vi "ref_Wrist_imp_PYBR_CH_v9.vi"() -> ()   [LabVIEW 2017]
uses:
  <vilib>/rvi/FXPMathLib/FxpSinAndCos/subVIs/nifxpmath_SinAndCos_SimConfig.ctl
  <vilib>/rvi/Emulation/niFpgaGetClockAttributes.vi
  <vilib>/rvi/Emulation/niFpgaSctlEmulationGetInTimedLoop.vi
  <vilib>/rvi/Emulation/niFpgaEmulationReportErrorSimple.vi
  <vilib>/rvi/eio/common/nirviEmuTemplateMethod_errors.vi
  <vilib>/rvi/Emulation/niFpgaProcessEmulError.vi
  <vilib>/rvi/Emulation/niFpgaCriticalErrorInLSC.vi
  <vilib>/rvi/interface/RandomDataEmulation/nirviRandomDataMultiElementFPGAFIFO.vi
  <instcachedir>/0/nirviRandomDataMultiElementFPGAFIFO_6740B454F3C245F78F76ED91F73FD8DB.lvgen/nirviRandomDataMultiElementFPGAFIFO_6740B454F3C245F78F76ED91F73FD8DB_003.vi
  <vilib>/rvi/interface/RandomDataEmulation/niFpgaRandomDataHandleErrors.vi
  <vilib>/rvi/FXPMathLib/FxpSinAndCos/simVIs/DllFxpSinAndCosTemp_sub.vi
  <vilib>/eio/EIONode/EIONode.xnode
  <vilib>/rvi/FXPMathLib/FxpMul/XNode/nifxpmath_Multiplier.xnode
  <vilib>/rvi/FXPMathLib/FxpSub/XNode/nifxpmath_Sub.xnode
  <vilib>/rvi/FXPMathLib/FxpAdd/XNode/nifxpmath_Add.xnode
  <vilib>/rvi/DataTransferAndStorage/Container/XNode/niFpgaContainer.xnode
  <vilib>/rvi/interface/RandomDataEmulation/nirviRandomDataFpgaMultiElementTemplate.vi
  <vilib>/rvi/FXPMathLib/FxpSinAndCos/XNode/nifxpmath_SinAndCos.xnode
  <vilib>/rvi/Analysis/measure/butterworth/XNode/niFpgaButterworthFilter.xnode
  <vilib>/rvi/FXPMathLib/sim/FxpSim.dll
panel:
  in  "Start_two":bool=TRUE
  in  "FIFO":i16(ring) items=["Inverse", "Forward", "Elbow"]
  out "Db_e":fxp<+/-,26,11>
  in  "time stop b":fxp<+,64,32>=5.0 format="%#_42g"
  out "Forward/Backward (b)":bool
  in  "CASE (b)":i16(ring) caption="Numeric" items=["Backward", "Forward", "Original"]
  in  "Sin/Step (b)":i16(ring) items=["Step", "Sin"]
  in  "ATOM b\nVelocity method":i16(ring) items=["M_average", "T_method"]
  in  "Encoder b\nVelocity method":i16(ring) items=["M_average", "T_method"]
  in  "phase(rad/pi)_b":fxp<+/-,16,3>
  in  "ATOM (P/Y)\nVelocity Method":i16(ring) items=["M_Average", "T_method"]
  in  "Encoder (P/Y)\nVelocity Method":i16(ring) items=["M_average", "T_method"]
  out "Encoder Position_b":i32
  out "rad(NrTheta)_b":fxp<+/-,33,18> format="%.21g"
  out "Db(mm)":fxp<+/-,22,7>
  in  "Encoder Reset_b":bool
  out "vd_b_F":fxp<+/-,20,5>
  out "vq_b_F":fxp<+/-,20,5> format="%.57g"
  out "Fb_PID":fxp<+/-,21,11>
  in  "fb_tolerance":fxp<+,32,9>=1.0
  out "fb_tilde":fxp<+/-,21,11>
  in  "Kpb":fxp<+,11,7>=0.375
  in  "Kib":fxp<+,27,10>
  in  "Kdb":fxp<+,26,2>
  out "fbt_i":fxp<+/-,32,9>
  out "dFb_PID":fxp<+/-,25,15>
  in  "scaled coe_dFb_PID":i32[](array[numeric])=[1067016412, 3362706]
  out "Db_dd":fxp<+/-,25,15>
  in  "scaled coe_Db_dd":i32[](array[numeric])=[1067016412, 3362706]
  out "xb_dd":fxp<+/-,25,15>
  in  "scaled coe_xb_dd":i32[](array[numeric])=[1067016412, 3362706]
  in  "kb":fxp<+,15,8>
  out "xb(mm)":fxp<+/-,22,7>
  out "fb":fxp<+/-,20,10>
  in  "Atom Reset_b":bool
  out "Atom_Position_b":i32
  out "Sin wave time (s) b":fxp<+,64,32>
  out "Db_d(mm/s)":fxp<+/-,32,12>
  out "Omega_b(rad/s)":fxp<+/-,32,18>
  in  "xb_d_M_avg_Tc (uSec)":u32 caption="M_avg_Tc (uSec)"
  out "xb_d(M_avg method)":fxp<+/-,25,10>
  out "vb_b":fxp<+/-,20,5> format="%.21g"
  out "va_b":fxp<+/-,20,5> format="%.21g"
  in  "Stop Motor_b":bool
  out "Dabr_sin/cos":fxp<+/-,22,8>
  in  "Sin_offset_b":fxp<+/-,16,5>
  in  "Sin_mag_b":fxp<+/-,17,6>
  out "Dabr_d":fxp<+/-,33,10>
  out "Dabr_dd":fxp<+/-,34,12>
  in  "Sin_freq_b (Hz)":fxp<+,16,3>
  out "fbr":fxp<+/-,20,10>
  in  "Kvb":fxp<+,15,8>
  in  "Bvb":fxp<+,15,8>
  in  "Dbr":fxp<+/-,22,8>
  out "Step/Sin Db":bool
  out "fbt_d":fxp<+/-,25,15>
  out "Dab_ed":fxp<+/-,33,10>
  out "Dab_edd":fxp<+/-,34,12>
  out "xb_d(mm/s)":fxp<+/-,25,10>
  in  "Db_d_M_avg_Tc (uSec)":u32 caption="M_avg_Tc (uSec)"
  out "Omega_b(M_avg)":fxp<+/-,32,18>
  out "Db_d(M_avg method)":fxp<+/-,32,12>
  in  "fb_lmpact":fxp<+,16,11>
  in  "Step / Sin (py)":i16(ring) items=["Step", "Sin"]
  in  "CASE (py)":i16(ring) caption="Numeric" items=["Backward", "Forward", "Original"]
  out "Dyr_sin/cos":fxp<+/-,24,10>
  in  "Sin_offset_y1":fxp<+/-,16,5>
  in  "Sin_mag_y1":fxp<+/-,17,6>
  out "Dyr_d":fxp<+/-,35,12>
  out "Dyr_dd":fxp<+/-,36,14>
  in  "Sin_freq(Hz)_y1":fxp<+,16,3>
  in  "phase(rad/pi)_y1":fxp<+/-,16,3>
  in  "Sin_offset_y2":fxp<+/-,16,5>
  in  "Sin_mag_y2":fxp<+/-,17,6>
  in  "Sin_freq(Hz)_y2":fxp<+,16,3>
  in  "phase(rad/pi)_y2":fxp<+/-,16,3>
  in  "Sin_offset_y3":fxp<+/-,16,5>
  in  "Sin_mag_y3":fxp<+/-,17,6>
  in  "Sin_freq(Hz)_y3":fxp<+,16,3>
  in  "phase(rad/pi)_y3":fxp<+/-,16,3>
  out "Dy_ed":fxp<+/-,33,10>
  out "Dy_edd":fxp<+/-,34,12>
  out "fyt_d":fxp<+/-,25,15>
  in  "ky":fxp<+,15,8>
  out "Dy_d(mm/s)":fxp<+/-,32,12>
  out "Omega_y(rad/s)":fxp<+/-,32,18>
  out "xy_d(mm/s)":fxp<+/-,25,10>
  out "xy_d(M_avg)":fxp<+/-,25,10>
  out "Omega_y(M_avg)":fxp<+/-,32,18>
  out "Dy_d(M_avg)":fxp<+/-,32,12>
  out "Encoder Position_y":i32
  out "rad(NrTheta)_y":fxp<+/-,33,18> format="%.21g"
  out "Dy(mm)":fxp<+/-,22,7>
  out "vd_y_F":fxp<+/-,20,5>
  out "vq_y_F":fxp<+/-,20,5> format="%.57g"
  out "Fy_PID":fxp<+/-,21,11>
  in  "fy_tolerance":fxp<+,32,9>=1.0
  out "fy_tilde":fxp<+/-,21,11>
  in  "Kpy":fxp<+,11,7>=0.375
  in  "Kiy":fxp<+,27,10>
  in  "Kdy":fxp<+,26,2>
  out "fyt_i":fxp<+/-,32,9>
  out "dFy_PID":fxp<+/-,25,15>
  out "Dy_dd":fxp<+/-,25,15>
  out "xy_dd":fxp<+/-,25,15>
  out "xy(mm)":fxp<+/-,22,7>
  out "fy":fxp<+/-,20,10>
  out "Atom_Position_y":i32
  out "vb_y":fxp<+/-,20,5> format="%.21g"
  out "va_y":fxp<+/-,20,5> format="%.21g"
  out "fyr":fxp<+/-,20,10>
  in  "Kvy":fxp<+,15,8>
  in  "Bvy":fxp<+,10,3>
  out "Dy_e":fxp<+/-,26,11>
  in  "Dyr":fxp<+/-,22,8>
  out "Forward/Backward (py)":bool
  in  "time stop py":fxp<+,64,32>=5.0 format="%#_42g"
  in  "Sin_offset_p3":fxp<+/-,16,5>
  in  "Sin_mag_p3":fxp<+/-,17,6>
  in  "Sin_freq(Hz)_p3":fxp<+,16,3>
  in  "phase(rad/pi)_p3":fxp<+/-,16,3>
  in  "Sin_offset_p2":fxp<+/-,16,5>
  in  "Sin_mag_p2":fxp<+/-,17,6>
  in  "Sin_freq(Hz)_p2":fxp<+,16,3>
  in  "phase(rad/pi)_p2":fxp<+/-,16,3>
  in  "phase(rad/pi)_p1":fxp<+/-,16,3>
  in  "fpy_Impact":fxp<+,16,11>
  in  "Dpy_d_M_avg_Tc (uSec)":u32 caption="M_avg_Tc (uSec)"
  out "Omega_p(rad/s)":fxp<+/-,32,18>
  out "Omega_p(M_avg)":fxp<+/-,32,18>
  out "xp_dd":fxp<+/-,25,15>
  in  "scaled coe_xpy_dd":i32[](array[numeric])=[1067016412, 3362706]
  out "Dp_dd":fxp<+/-,25,15>
  in  "scaled coe_Dpy_dd":i32[](array[numeric])=[1067016412, 3362706]
  out "Dp_edd":fxp<+/-,34,12>
  out "Dp_ed":fxp<+/-,33,10>
  out "fpr":fxp<+/-,20,10>
  in  "Kvp":fxp<+,15,8>
  in  "Bvp":fxp<+,10,3>
  out "Dp_e":fxp<+/-,26,11>
  in  "Dpr":fxp<+/-,22,8>
  out "Step/Sin Dpy":bool
  out "Dpr_sin/cos":fxp<+/-,24,10>
  in  "Sin_offset_p1":fxp<+/-,16,5>
  in  "Sin_mag_p1":fxp<+/-,17,6>
  out "Dpr_d":fxp<+/-,35,12>
  out "Dpr_dd":fxp<+/-,36,14> format="%.26g"
  in  "Sin_freq(Hz)_p1":fxp<+,16,3>
  out "Dp_d(M_avg)":fxp<+/-,32,12>
  out "xp_d(M_avg)":fxp<+/-,25,10>
  in  "xpy_d_M_avg_Tc (uSec)":u32 caption="M_avg_Tc (uSec)"
  out "fpt_d":fxp<+/-,25,15>
  out "Dp_d(mm/s)":fxp<+/-,32,12>
  out "Atom_Position_p":i32
  out "xp_d(mm/s)":fxp<+/-,25,10>
  in  "dFb_PID_add":bool
  in  "scaled coe_dFpy_PID":i32[](array[numeric])=[1067016412, 3362706]
  out "dFp_PID":fxp<+/-,25,15>
  out "Sin wave time (s)":fxp<+,64,32>
  in  "Atom Reset":bool
  out "xp(mm)":fxp<+/-,22,7>
  in  "Coe Ini":bool
  in  "Encoder Reset":bool
  in  "Stop Motor":bool
  in  "Kip":fxp<+,27,10>
  in  "Kdp":fxp<+,26,2>
  out "fpt_i":fxp<+/-,32,9>
  in  "Kpp":fxp<+,11,7>=0.375
  in  "kp":fxp<+,15,8>
  out "fp":fxp<+/-,20,10>
  out "fp_tilde":fxp<+/-,21,11>
  out "Fp_PID":fxp<+/-,21,11>
  in  "fp_tolerance":fxp<+,32,9>=1.0
  out "Encoder Position_p":i32
  out "rad(NrTheta)_p":fxp<+/-,33,18> format="%.21g"
  out "Dp(mm)":fxp<+/-,22,7>
  out "vq_p_F":fxp<+/-,20,5> format="%.57g"
  out "vd_p_F":fxp<+/-,20,5>
  out "va_p":fxp<+/-,20,5> format="%.21g"
  out "vb_p":fxp<+/-,20,5> format="%.21g"
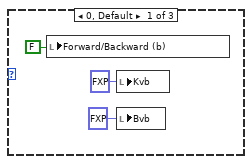
[diagram p4: hidden frame]
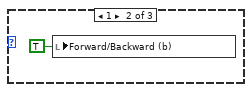
[diagram p5: hidden frame]
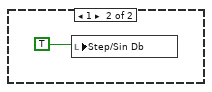
[diagram p6: hidden frame]
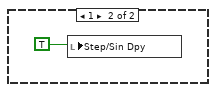
[diagram p7: hidden frame]
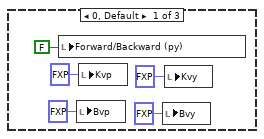
[diagram p8: hidden frame]
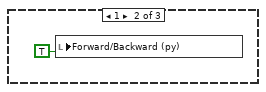
[diagram p9: hidden frame]
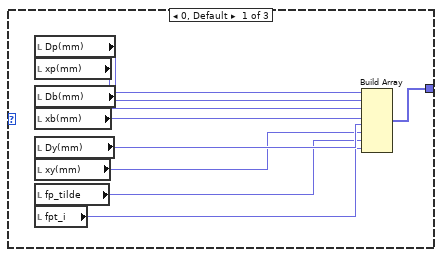
[diagram p20: hidden frame]
diagram:
  w2 = FALSE ("Encoder Reset_b")
  w11 = 25  # M_avg_n
  w7 = 25  # M_avg_n
  w21 = 25  # M_avg_n
  w17 = 25  # M_avg_n
  w1 = FALSE ("Atom Reset_b")
  w5 = TRUE ("Stop Motor_b")
  w26 = 25  # M_avg_n
  w30 = 25  # M_avg_n
  n1 = for {
    N: w11 -> [_]
    tunnel: [w34] -> w13 mode=indexing
    tunnel: [w32] -> w12 mode=indexing
    tunnel: ["Db_d_M_avg_Tc (uSec)"] -> w10
    n2 = local read "Encoder Position_b"() -> (w32:i32)
    n3 = call "Wait11"("Count(uSec)"="Db_d_M_avg_Tc (uSec)") -> ("Tick Count(uSec)"=w34:u32)
  }
  n4 = for {
    N: w7 -> [_]
    tunnel: [w37] -> w6 mode=indexing
    tunnel: ["xb_d_M_avg_Tc (uSec)"] -> w8
    tunnel: [w35] -> w9 mode=indexing
    n5 = local read "Atom_Position_b"() -> (w35:i32)
    n6 = call "Wait9"("Count(uSec)"="xb_d_M_avg_Tc (uSec)") -> ("Tick Count(uSec)"=w37:u32)
  }
  n7 = while "Db_d(M_avg method)" {
    shift-right: [w48] -> _
    shift-left: w13 -> [w51]
    tunnel: w11 -> [w49]
    shift-right: [w46] -> _
    shift-left: w12 -> [w44]
    shift-right: [w39] -> _
    shift-left: _ -> [w42]
    tunnel: w10 -> [w41]
    stop <- FALSE stop-if-true
    n8 = Index Array(array=w51, index=0) -> (element=w47:u32)
    n9 = Multiply(x=w49, y=w41) -> (x*y=w54:u32)
    n10 = Index Array(array=w44, index=0) -> (element=w43:i32)
    n11 = Add(x=w54, y=w47) -> (x+y=w53:u32)
    n12 = call "Tick Count20"() -> ("Tick Count(uSec)"=w50:u32)
    n13 = Greater Or Equal?(x=w50, y=w53) -> (x >= y?=w52:bool)
    n14 = case shown="True" w52 {
      tunnel: w51 -> [w59 w81]
      tunnel: w50 -> [_ w75]
      tunnel: w49 -> [_ w64]
      tunnel: [w59 w77] -> w48
      tunnel: w47 -> [_ w76]
      tunnel: w44 -> [w58 w65]
      tunnel: [w58 w63] -> w46
      tunnel: [w57 w62] -> w39
      tunnel: w43 -> [_ w60]
      tunnel: w42 -> [w57 _]
      frame False {
      }
      frame True {
        n15 = local read "Encoder Position_b"() -> (w69:i32)
        n16 = Subtract(x=w75, y=w76) -> (x-y=w74:u32)
        n17 = To Fixed-Point(number=w74) -> (fixed-point=w61:fxp<+,32,32>)  [unwired: 1 in]
        n18 = Insert Into Array(array=w81, index=w64, new element=w75) -> (w80:u32[])
        n19 = Insert Into Array(array=w65, index=w64, new element=w69) -> (w66:i32[])
        n20 = Subtract(x=w69, y=w60) -> (x-y=w70:i32)
        n21 = Multiply(x=w70, y=2500) -> (x*y=w72:i32)
        n22 = Delete From Array(array=w80, length=1, index=0) -> (array with subset deleted=w77:u32[])  [unwired: 1 out]
        n23 = Delete From Array(array=w66, length=1, index=0) -> (array with subset deleted=w63:i32[])  [unwired: 1 out]
        n24 = To Fixed-Point(number=w72) -> (fixed-point=w73:fxp<+/-,32,32>)  [unwired: 1 in]
        n25 = Divide(x=w73, y=w61) -> (x/y=w62:fxp<+/-,32,12>)
      }
    }
    "Db_d(M_avg method)" <- w39
    n26 = Multiply(x=w39, y=fxp<+/-,32,12> 3.1415929794311523 ("x")) -> (x*y=→"Omega_b(M_avg)":fxp<+/-,32,18>)
  }
  n27 = while "M_avg method" {
    shift-right: [w89] -> _
    shift-left: w6 -> [w92]
    shift-right: [w83] -> _
    shift-left: w9 -> [w86]
    tunnel: w7 -> [w90]
    shift-right: [w85] -> _
    shift-left: _ -> [w84]
    tunnel: w8 -> [w82]
    stop <- FALSE stop-if-true
    n28 = Index Array(array=w92, index=0) -> (element=w88:u32)
    n29 = Multiply(x=w90, y=w82) -> (x*y=w95:u32)
    n30 = Index Array(array=w86, index=0) -> (element=w87:i32)
    n31 = Add(x=w95, y=w88) -> (x+y=w94:u32)
    n32 = call "Tick Count18"() -> ("Tick Count(uSec)"=w91:u32)
    n33 = Greater Or Equal?(x=w91, y=w94) -> (x >= y?=w93:bool)
    n34 = case shown="True" w93 {
      tunnel: w92 -> [w101 w123]
      tunnel: w91 -> [_ w117]
      tunnel: w90 -> [_ w103]
      tunnel: [w101 w119] -> w89
      tunnel: w88 -> [_ w118]
      tunnel: w86 -> [w100 w114]
      tunnel: w87 -> [_ w110]
      tunnel: [w99 w105] -> w85
      tunnel: w84 -> [w99 _]
      tunnel: [w100 w104] -> w83
      frame False {
      }
      frame True {
        n35 = local read "Atom_Position_b"() -> (w111:i32)
        n36 = Subtract(x=w117, y=w118) -> (x-y=w116:u32)
        n37 = To Fixed-Point(number=w116) -> (fixed-point=w102:fxp<+,32,32>)  [unwired: 1 in]
        n38 = Insert Into Array(array=w123, index=w103, new element=w117) -> (w122:u32[])
        n39 = Insert Into Array(array=w114, index=w103, new element=w111) -> (w115:i32[])
        n40 = Subtract(x=w111, y=w110) -> (x-y=w109:i32)
        n41 = Multiply(x=w109, y=-1000) -> (x*y=w107:i32)
        n42 = Delete From Array(array=w122, length=1, index=0) -> (array with subset deleted=w119:u32[])  [unwired: 1 out]
        n43 = Delete From Array(array=w115, length=1, index=0) -> (array with subset deleted=w104:i32[])  [unwired: 1 out]
        n44 = To Fixed-Point(number=w107) -> (fixed-point=w106:fxp<+/-,32,32>)  [unwired: 1 in]
        n45 = Divide(x=w106, y=w102) -> (x/y=w105:fxp<+/-,25,10>)
      }
    }
    "xb_d(M_avg method)" <- w85
  }
  n46 = while "Encoder_b" {
    shift-right: [w125] -> _
    shift-left: _ -> [w137]
    shift-right: [w124] -> _
    shift-left: _ -> [w136]
    shift-right: [w129] -> _
    shift-left: _ -> [w135]
    stop <- FALSE stop-if-true
    n47 = xnode "FPGA I/O Node"() -> ("Mod4/DI3"=w127:bool, "Mod4/DI4"=w126:bool)  [unwired: 2 in, 2 out]
    n48 = call "encoder_sub.vi"("A_pre"=w137, "B_pre"=w136, "Encoder Position_pre"=w135, "A input"=w127, "Encoder Position Reset"="Encoder Reset_b", "B input"=w126) -> ("A"=w125:bool, "B"=w124:bool, "Encoder Position (Counts)"=w129:i32)  [unwired: 19 in]
    "Encoder Position_b" <- w129
    n49 = To Fixed-Point(number=w129) -> (fixed-point=w132:fxp<+/-,18,18>)  [unwired: 1 in]
    n50 = xnode ("High Throughput Multiply")("x"=w132, "y"=fxp<+/-,15,-7> 0.0012500286102294922) -> ("x*y"=→"Db(mm)":fxp<+/-,22,7>)
    n51 = xnode ("High Throughput Multiply")("x"=w132, "y"=fxp<+,24,0> 0.125) -> ("x*y"=→"rad(NrTheta)_b":fxp<+/-,33,18>)
  }
  n52 = while "Atom_b" {
    shift-right: [w152] -> _
    shift-left: _ -> [w150]
    shift-right: [w151] -> _
    shift-left: _ -> [w149]
    shift-right: [w140] -> _
    shift-left: _ -> [w146]
    stop <- FALSE stop-if-true
    n53 = xnode "FPGA I/O Node"() -> ("Mod4/DI0"=w148:bool, "Mod4/DI1"=w147:bool)  [unwired: 2 in, 2 out]
    n54 = call "encoder_sub.vi"("A_pre"=w150, "B_pre"=w149, "Encoder Position_pre"=w146, "A input"=w148, "Encoder Position Reset"="Atom Reset_b", "B input"=w147) -> ("A"=w152:bool, "B"=w151:bool, "Encoder Position (Counts)"=w140:i32)  [unwired: 19 in]
    "Atom_Position_b" <- w140
    n55 = To Fixed-Point(number=w140) -> (fixed-point=w144:fxp<+/-,18,18>)  [unwired: 1 in]
    n56 = xnode ("High Throughput Multiply")("x"=w144, "y"=fxp<+/-,20,-5> -0.0009999871253967285) -> ("x*y"=w142:fxp<+/-,22,7>)
    "xb(mm)" <- w142
    n57 = Multiply(x=w142, y="kb") -> (x*y=→"fb":fxp<+/-,20,10>)
  }
  n58 = for {
    N: w21 -> [_]
    tunnel: [w156] -> w23 mode=indexing
    tunnel: [w155] -> w22 mode=indexing
    tunnel: [w154] -> w20
    n59 = local read "Dpy_d_M_avg_Tc (uSec)"() -> (w154:u32)
    n60 = local read "Encoder Position_y"() -> (w155:i32)
    n61 = call "Wait7"("Count(uSec)"=w154) -> ("Tick Count(uSec)"=w156:u32)
  }
  n62 = for {
    N: w17 -> [_]
    tunnel: [w159] -> w16 mode=indexing
    tunnel: [w157] -> w18
    tunnel: [w158] -> w19 mode=indexing
    n63 = local read "xpy_d_M_avg_Tc (uSec)"() -> (w157:u32)
    n64 = local read "Atom_Position_y"() -> (w158:i32)
    n65 = call "Wait6"("Count(uSec)"=w157) -> ("Tick Count(uSec)"=w159:u32)
  }
  n66 = for {
    N: w26 -> [_]
    tunnel: [w162] -> w24 mode=indexing
    tunnel: [w160] -> w25 mode=indexing
    tunnel: ["Dpy_d_M_avg_Tc (uSec)"] -> w27
    n67 = local read "Encoder Position_p"() -> (w160:i32)
    n68 = call "Wait4"("Count(uSec)"="Dpy_d_M_avg_Tc (uSec)") -> ("Tick Count(uSec)"=w162:u32)
  }
  n69 = for {
    N: w30 -> [_]
    tunnel: [w165] -> w31 mode=indexing
    tunnel: ["xpy_d_M_avg_Tc (uSec)"] -> w29
    tunnel: [w163] -> w28 mode=indexing
    n70 = local read "Atom_Position_p"() -> (w163:i32)
    n71 = call "Wait3"("Count(uSec)"="xpy_d_M_avg_Tc (uSec)") -> ("Tick Count(uSec)"=w165:u32)
  }
  n72 = while "PID force controller_imp_p" {
    stop <- FALSE stop-if-true
    n73 = flat-sequence {
      tunnel: [w169] -> w166
      tunnel: [w184] -> w167
      tunnel: w166 -> [w183]
      tunnel: w167 -> [w201]
      frame #0 {
        # "SEA imp position controller_p"
        n74 = local read "Step/Sin Dpy"() -> (w182:bool)
        n75 = local read "Dpr_sin/cos"() -> (w181:fxp<+/-,24,10>)
        n76 = local read "Dp(mm)"() -> (w174:fxp<+/-,22,7>)
        n77 = local read "xp(mm)"() -> (w173:fxp<+/-,22,7>)
        n78 = local read "Dp_ed"() -> (w176:fxp<+/-,33,10>)
        n79 = Select(t=w181, s=w182, f="Dpr") -> (s? t:f=w179:fxp<+/-,24,10>)
        n80 = Subtract(x=w174, y=w173) -> (x-y=w175:fxp<+/-,22,7>)
        n81 = Subtract(x=w179, y=w175) -> (x-y=w170:fxp<+/-,25,10>)
        "Dp_e" <- w170
        n82 = Multiply(x=w170, y="Kvp") -> (x*y=w172:fxp<+/-,40,18>)
        n83 = Multiply(x=w176, y="Bvp") -> (x*y=w171:fxp<+/-,43,13>)
        n84 = Add(x=w172, y=w171) -> (x+y=w169:fxp<+/-,20,10>)
        "fpr" <- w169
      }
      frame #1 {
        # "PID force controller_imp_p"
        n85 = local read "fp"() -> (w195:fxp<+/-,20,10>)
        n86 = local read "fpt_d"() -> (w186:fxp<+/-,25,15>)
        n87 = xnode "High Throughput Subtract"("x"=w183, "y"=w195) -> ("x-y"=w197:fxp<+/-,21,11>)
        "fp_tilde" <- w197
        n88 = local read "fpt_i"() -> (w193:fxp<+/-,32,9>)
        n89 = Absolute Value(x=w197) -> (abs(x)=w199:fxp<+,21,11>)
        n90 = xnode ("High Throughput Multiply")("x"="Kpp", "y"=w197) -> ("x*y"=w196:fxp<+/-,33,17>)
        n91 = xnode ("High Throughput Multiply")("x"="Kdp", "y"=w186) -> ("x*y"=w190:fxp<+/-,31,21>)
        n92 = xnode ("High Throughput Add")("x"=w196, "y"=w190) -> ("x+y"=w194:fxp<+/-,21,11>)
        n93 = xnode ("High Throughput Multiply")("x"="Kip", "y"=w193) -> ("x*y"=w192:fxp<+/-,31,14>)
        n94 = Greater?(x=w199, y="fp_tolerance") -> (0:w198:bool)
        n95 = xnode ("High Throughput Add")("x"=w194, "y"=w192) -> ("x+y"=w191:fxp<+/-,21,11>)
        n96 = Select(t=w191, s=w198, f=fxp<+/-,21,11> 0.0) -> (s? t:f=w184:fxp<+/-,21,11>)
        "Fp_PID" <- w184
      }
      frame #2 {
        w204 = fxp<+,3,2> 0.5  # belt_coe
        # "Quadrature drive_p"
        n97 = local read "Omega_p(rad/s)"() -> (w206:fxp<+/-,32,18>)
        n98 = local read "dFp_PID"() -> (w210:fxp<+/-,25,15>)
        n99 = Select(t=fxp<+/-,25,15> 0.0 ("f"), s="dFb_PID_add", f=w210) -> (s? t:f=w207:fxp<+/-,25,15>)
        n100 = Multiply(x=w204, y=w201) -> (x*y=w205:fxp<+/-,24,13>)
        n101 = call "Oriental_step_motor_PKP214D06A.vi"("F_Threshold"=fxp<+,12,12> 10.0, "dFmr"=w207, "omega"=w206, "Fmr"=w205) -> ("vq_F"=→"vq_p_F":fxp<+/-,20,5>, "vd_F"=→"vd_p_F":fxp<+/-,20,5>)  [unwired: 6 in]
      }
    }
  }
  n102 = while "PID force controller_imp_y" {
    stop <- FALSE stop-if-true
    n103 = flat-sequence {
      tunnel: [w215] -> w213
      tunnel: w213 -> [w230]
      tunnel: [w229] -> w212
      tunnel: w212 -> [w247]
      frame #0 {
        # "SEA imp position controller_y"
        n104 = local read "Step/Sin Dpy"() -> (w216:bool)
        n105 = local read "Dyr_sin/cos"() -> (w217:fxp<+/-,24,10>)
        n106 = local read "Dy(mm)"() -> (w224:fxp<+/-,22,7>)
        n107 = local read "xy(mm)"() -> (w225:fxp<+/-,22,7>)
        n108 = local read "Dp_ed"() -> (w222:fxp<+/-,33,10>)
        n109 = Select(t=w217, s=w216, f="Dyr") -> (s? t:f=w219:fxp<+/-,24,10>)
        n110 = Subtract(x=w224, y=w225) -> (x-y=w223:fxp<+/-,22,7>)
        n111 = Subtract(x=w219, y=w223) -> (x-y=w228:fxp<+/-,25,10>)
        "Dy_e" <- w228
        n112 = Multiply(x=w228, y="Kvy") -> (x*y=w226:fxp<+/-,40,18>)
        n113 = Multiply(x=w222, y="Bvy") -> (x*y=w227:fxp<+/-,43,13>)
        n114 = Add(x=w226, y=w227) -> (x+y=w215:fxp<+/-,20,10>)
        "fyr" <- w215
      }
      frame #1 {
        # "PID force controller_imp_y"
        n115 = local read "fy"() -> (w241:fxp<+/-,20,10>)
        n116 = local read "fyt_d"() -> (w232:fxp<+/-,25,15>)
        n117 = xnode "High Throughput Subtract"("x"=w230, "y"=w241) -> ("x-y"=w243:fxp<+/-,21,11>)
        "fy_tilde" <- w243
        n118 = local read "fyt_i"() -> (w239:fxp<+/-,32,9>)
        n119 = Absolute Value(x=w243) -> (abs(x)=w245:fxp<+,21,11>)
        n120 = xnode ("High Throughput Multiply")("x"="Kpy", "y"=w243) -> ("x*y"=w242:fxp<+/-,33,17>)
        n121 = xnode ("High Throughput Multiply")("x"="Kdy", "y"=w232) -> ("x*y"=w236:fxp<+/-,31,21>)
        n122 = xnode ("High Throughput Add")("x"=w242, "y"=w236) -> ("x+y"=w240:fxp<+/-,21,11>)
        n123 = xnode ("High Throughput Multiply")("x"="Kiy", "y"=w239) -> ("x*y"=w238:fxp<+/-,31,14>)
        n124 = Greater?(x=w245, y="fy_tolerance") -> (0:w244:bool)
        n125 = xnode ("High Throughput Add")("x"=w240, "y"=w238) -> ("x+y"=w237:fxp<+/-,21,11>)
        n126 = Select(t=w237, s=w244, f=fxp<+/-,21,11> 0.0) -> (s? t:f=w229:fxp<+/-,21,11>)
        "Fy_PID" <- w229
      }
      frame #2 {
        w250 = fxp<+,3,2> 0.5  # belt_coe
        # "Quadrature drive_y"
        n127 = local read "dFb_PID_add"() -> (w257:bool)
        n128 = local read "Omega_y(rad/s)"() -> (w255:fxp<+/-,32,18>)
        n129 = local read "dFy_PID"() -> (w251:fxp<+/-,25,15>)
        n130 = Select(t=fxp<+/-,25,15> 0.0 ("f"), s=w257, f=w251) -> (s? t:f=w254:fxp<+/-,25,15>)
        n131 = Multiply(x=w250, y=w247) -> (x*y=w256:fxp<+/-,24,13>)
        n132 = call "Oriental_step_motor_PKP214D06A.vi"("F_Threshold"=fxp<+,12,12> 10.0, "dFmr"=w254, "omega"=w255, "Fmr"=w256) -> ("vq_F"=→"vq_y_F":fxp<+/-,20,5>, "vd_F"=→"vd_y_F":fxp<+/-,20,5>)  [unwired: 6 in]
      }
    }
  }
  n133 = while "PID force controller_imp_b" {
    stop <- FALSE stop-if-true
    n134 = flat-sequence {
      tunnel: [w261] -> w258
      tunnel: [w276] -> w259
      tunnel: w258 -> [w275]
      tunnel: w259 -> [w293]
      frame #0 {
        # "SEA imp position controller_b"
        n135 = local read "Step/Sin Db"() -> (w273:bool)
        n136 = local read "Dabr_sin/cos"() -> (w272:fxp<+/-,22,8>)
        n137 = local read "Db(mm)"() -> (w265:fxp<+/-,22,7>)
        n138 = local read "xb(mm)"() -> (w264:fxp<+/-,22,7>)
        n139 = local read "Dab_ed"() -> (w267:fxp<+/-,33,10>)
        n140 = Select(t=w272, s=w273, f="Dbr") -> (s? t:f=w270:fxp<+/-,22,8>)
        n141 = Subtract(x=w265, y=w264) -> (x-y=w266:fxp<+/-,22,7>)
        n142 = Subtract(x=w270, y=w266) -> (x-y=w274:fxp<+/-,24,9>)
        "Db_e" <- w274
        n143 = Multiply(x=w274, y="Kvb") -> (x*y=w263:fxp<+/-,39,17>)
        n144 = Multiply(x=w267, y="Bvb") -> (x*y=w262:fxp<+/-,48,18>)
        n145 = Add(x=w263, y=w262) -> (x+y=w261:fxp<+/-,20,10>)
        "fbr" <- w261
      }
      frame #1 {
        # "PID force controller_imp_b"
        n146 = local read "fb"() -> (w287:fxp<+/-,20,10>)
        n147 = local read "fbt_d"() -> (w278:fxp<+/-,25,15>)
        n148 = xnode "High Throughput Subtract"("x"=w275, "y"=w287) -> ("x-y"=w289:fxp<+/-,21,11>)
        "fb_tilde" <- w289
        n149 = local read "fbt_i"() -> (w285:fxp<+/-,32,9>)
        n150 = Absolute Value(x=w289) -> (abs(x)=w291:fxp<+,21,11>)
        n151 = xnode ("High Throughput Multiply")("x"="Kpb", "y"=w289) -> ("x*y"=w288:fxp<+/-,33,17>)
        n152 = xnode ("High Throughput Multiply")("x"="Kdb", "y"=w278) -> ("x*y"=w282:fxp<+/-,31,21>)
        n153 = xnode ("High Throughput Add")("x"=w288, "y"=w282) -> ("x+y"=w286:fxp<+/-,21,11>)
        n154 = xnode ("High Throughput Multiply")("x"="Kib", "y"=w285) -> ("x*y"=w284:fxp<+/-,31,14>)
        n155 = Greater?(x=w291, y="fb_tolerance") -> (0:w290:bool)
        n156 = xnode ("High Throughput Add")("x"=w286, "y"=w284) -> ("x+y"=w283:fxp<+/-,21,11>)
        n157 = Select(t=w283, s=w290, f=fxp<+/-,21,11> 0.0) -> (s? t:f=w276:fxp<+/-,21,11>)
        "Fb_PID" <- w276
      }
      frame #2 {
        # "Quadrature drive_b"
        n158 = local read "dFb_PID_add"() -> (w301:bool)
        n159 = local read "Omega_b(rad/s)"() -> (w299:fxp<+/-,32,18>)
        n160 = local read "dFb_PID"() -> (w296:fxp<+/-,25,15>)
        n161 = Select(t=fxp<+/-,25,15> 0.0 ("f"), s=w301, f=w296) -> (s? t:f=w300:fxp<+/-,25,15>)
        n162 = call "Oriental_step_motor_PKP225.vi"("F_Threshold"=fxp<+,12,12> 10.0, "dFmr"=w300, "omega"=w299, "Fmr"=w293) -> ("vq_F"=→"vq_b_F":fxp<+/-,20,5>, "vd_F"=→"vd_b_F":fxp<+/-,20,5>)  [unwired: 6 in]
      }
    }
  }
  n163 = while "AO_p" {
    stop <- FALSE stop-if-true
    n164 = flat-sequence {
      tunnel: [w306] -> w303
      tunnel: [w305] -> w302
      tunnel: w303 -> [w353]
      tunnel: w302 -> [w352]
      frame #0 {
        w313 = fxp<+/-,20,5> 0.0  # vq_p
        w312 = fxp<+/-,20,5> 0.0  # vd_p
        # "DQ Trans."
        n165 = local read "rad(NrTheta)_p"() -> (w321:fxp<+/-,33,18>)
        n166 = local read "vq_p_F"() -> (w310:fxp<+/-,20,5>)
        n167 = Select(t=w313, s="Stop Motor", f=w310) -> (s? t:f=w307:fxp<+/-,20,5>)
        n168 = local read "vd_p_F"() -> (w311:fxp<+/-,20,5>)
        n169 = xnode "High Throughput Sine & Cosine"("x (pi)"=w321) -> ("sin(x)"=w314:fxp<+/-,17,2>, "cos(x)"=w315:fxp<+/-,17,2>)
        n170 = Select(t=w312, s="Stop Motor", f=w311) -> (s? t:f=w308:fxp<+/-,20,5>)
        n171 = Negate(x=w307) -> (-x=w320:fxp<+/-,21,6>)
        n172 = Multiply(x=w308, y=w314) -> (x*y=w317:fxp<+/-,20,5>)
        n173 = Multiply(x=w308, y=w315) -> (x*y=w319:fxp<+/-,20,5>)
        n174 = Multiply(x=w307, y=w315) -> (x*y=w316:fxp<+/-,20,5>)
        n175 = Multiply(x=w320, y=w314) -> (x*y=w318:fxp<+/-,20,5>)
        n176 = Add(x=w316, y=w317) -> (x+y=w305:fxp<+/-,20,5>)
        "vb_p" <- w305
        n177 = Add(x=w319, y=w318) -> (x+y=w306:fxp<+/-,20,5>)
        "va_p" <- w306
      }
      frame #1 {
        # "AO"
        n178 = local read "Encoder Reset"() -> (w360:bool)
        n179 = Select(t=fxp<+/-,20,5> 3.0 ("Mod2/AO4"), s=w360, f=w353) -> (s? t:f=w358:fxp<+/-,20,5>)
        n180 = Select(t=fxp<+/-,20,5> 0.0 ("Mod2/AO4"), s=w360, f=w352) -> (s? t:f=w355:fxp<+/-,20,5>)
        n181 = Multiply(x=w358, y=fxp<+/-,20,5> -0.5) -> (x*y=w359:fxp<+/-,20,5>)
        n182 = Multiply(x=w355, y=fxp<+/-,20,5> -0.5) -> (x*y=w354:fxp<+/-,20,5>)
        n183 = xnode "FPGA I/O Node"("Mod2/AO0"=w359, "Mod2/AO1"=w354) -> ()  [unwired: 2 in, 2 out]
      }
    }
  }
  n184 = while "AO_y" {
    stop <- FALSE stop-if-true
    n185 = flat-sequence {
      tunnel: [w367] -> w364
      tunnel: [w366] -> w363
      tunnel: w364 -> [w414]
      tunnel: w363 -> [w413]
      frame #0 {
        w374 = fxp<+/-,20,5> 0.0  # vq_y
        w373 = fxp<+/-,20,5> 0.0  # vd_y
        # "DQ Trans."
        n186 = local read "rad(NrTheta)_y"() -> (w382:fxp<+/-,33,18>)
        n187 = local read "vq_y_F"() -> (w371:fxp<+/-,20,5>)
        n188 = local read "Stop Motor"() -> (w368:bool)
        n189 = Select(t=w374, s=w368, f=w371) -> (s? t:f=w369:fxp<+/-,20,5>)
        n190 = local read "vd_y_F"() -> (w372:fxp<+/-,20,5>)
        n191 = xnode "High Throughput Sine & Cosine"("x (pi)"=w382) -> ("sin(x)"=w375:fxp<+/-,17,2>, "cos(x)"=w376:fxp<+/-,17,2>)
        n192 = Select(t=w373, s=w368, f=w372) -> (s? t:f=w370:fxp<+/-,20,5>)
        n193 = Negate(x=w369) -> (-x=w381:fxp<+/-,21,6>)
        n194 = Multiply(x=w370, y=w375) -> (x*y=w378:fxp<+/-,20,5>)
        n195 = Multiply(x=w370, y=w376) -> (x*y=w380:fxp<+/-,20,5>)
        n196 = Multiply(x=w369, y=w376) -> (x*y=w377:fxp<+/-,20,5>)
        n197 = Multiply(x=w381, y=w375) -> (x*y=w379:fxp<+/-,20,5>)
        n198 = Add(x=w377, y=w378) -> (x+y=w366:fxp<+/-,20,5>)
        "vb_y" <- w366
        n199 = Add(x=w380, y=w379) -> (x+y=w367:fxp<+/-,20,5>)
        "va_y" <- w367
      }
      frame #1 {
        # "AO"
        n200 = local read "Encoder Reset"() -> (w421:bool)
        n201 = Select(t=fxp<+/-,20,5> 3.0 ("Mod2/AO4"), s=w421, f=w414) -> (s? t:f=w419:fxp<+/-,20,5>)
        n202 = Select(t=fxp<+/-,20,5> 0.0 ("Mod2/AO4"), s=w421, f=w413) -> (s? t:f=w416:fxp<+/-,20,5>)
        n203 = Multiply(x=w419, y=fxp<+/-,20,5> -0.5) -> (x*y=w420:fxp<+/-,20,5>)
        n204 = Multiply(x=w416, y=fxp<+/-,20,5> -0.5) -> (x*y=w415:fxp<+/-,20,5>)
        n205 = xnode "FPGA I/O Node"("Mod2/AO2"=w420, "Mod2/AO3"=w415) -> ()  [unwired: 2 in, 2 out]
      }
    }
  }
  n206 = while "AO_b" {
    stop <- FALSE stop-if-true
    n207 = flat-sequence {
      tunnel: [w428] -> w425
      tunnel: [w427] -> w424
      tunnel: w425 -> [w475]
      tunnel: w424 -> [w474]
      frame #0 {
        w435 = fxp<+/-,20,5> 0.0  # vq_b
        w434 = fxp<+/-,20,5> 0.0  # vd_b
        # "DQ Trans."
        n208 = local read "rad(NrTheta)_b"() -> (w443:fxp<+/-,33,18>)
        n209 = local read "vq_b_F"() -> (w432:fxp<+/-,20,5>)
        n210 = Select(t=w435, s="Stop Motor_b", f=w432) -> (s? t:f=w429:fxp<+/-,20,5>)
        n211 = local read "vd_b_F"() -> (w433:fxp<+/-,20,5>)
        n212 = xnode "High Throughput Sine & Cosine"("x (pi)"=w443) -> ("sin(x)"=w436:fxp<+/-,17,2>, "cos(x)"=w437:fxp<+/-,17,2>)
        n213 = Select(t=w434, s="Stop Motor_b", f=w433) -> (s? t:f=w430:fxp<+/-,20,5>)
        n214 = Negate(x=w429) -> (-x=w442:fxp<+/-,21,6>)
        n215 = Multiply(x=w430, y=w436) -> (x*y=w439:fxp<+/-,20,5>)
        n216 = Multiply(x=w430, y=w437) -> (x*y=w441:fxp<+/-,20,5>)
        n217 = Multiply(x=w429, y=w437) -> (x*y=w438:fxp<+/-,20,5>)
        n218 = Multiply(x=w442, y=w436) -> (x*y=w440:fxp<+/-,20,5>)
        n219 = Add(x=w438, y=w439) -> (x+y=w427:fxp<+/-,20,5>)
        "vb_b" <- w427
        n220 = Add(x=w441, y=w440) -> (x+y=w428:fxp<+/-,20,5>)
        "va_b" <- w428
      }
      frame #1 {
        # "AO"
        n221 = local read "Encoder Reset_b"() -> (w482:bool)
        n222 = Select(t=fxp<+/-,20,5> 3.0 ("Mod2/AO4"), s=w482, f=w475) -> (s? t:f=w480:fxp<+/-,20,5>)
        n223 = Select(t=fxp<+/-,20,5> 0.0 ("Mod2/AO4"), s=w482, f=w474) -> (s? t:f=w477:fxp<+/-,20,5>)
        n224 = Multiply(x=w480, y=fxp<+/-,20,5> -0.5) -> (x*y=w481:fxp<+/-,20,5>)
        n225 = Multiply(x=w477, y=fxp<+/-,20,5> -0.5) -> (x*y=w476:fxp<+/-,20,5>)
        n226 = xnode "FPGA I/O Node"("Mod2/AO4"=w481, "Mod2/AO5"=w476) -> ()  [unwired: 2 in, 2 out]
      }
    }
  }
  n227 = while "Encoder_p" {
    shift-right: [w486] -> _
    shift-left: _ -> [w498]
    shift-right: [w485] -> _
    shift-left: _ -> [w497]
    shift-right: [w490] -> _
    shift-left: _ -> [w496]
    stop <- FALSE stop-if-true
    n228 = xnode "FPGA I/O Node"() -> ("Mod5/DI3"=w488:bool, "Mod5/DI4"=w487:bool)  [unwired: 2 in, 2 out]
    n229 = call "encoder_sub.vi"("A_pre"=w498, "B_pre"=w497, "Encoder Position_pre"=w496, "A input"=w488, "Encoder Position Reset"="Encoder Reset", "B input"=w487) -> ("A"=w486:bool, "B"=w485:bool, "Encoder Position (Counts)"=w490:i32)  [unwired: 19 in]
    "Encoder Position_p" <- w490
    n230 = To Fixed-Point(number=w490) -> (fixed-point=w493:fxp<+/-,18,18>)  [unwired: 1 in]
    n231 = xnode ("High Throughput Multiply")("x"=w493, "y"=fxp<+/-,15,-7> 0.0012500286102294922) -> ("x*y"=→"Dp(mm)":fxp<+/-,22,7>)
    n232 = xnode ("High Throughput Multiply")("x"=w493, "y"=fxp<+,24,0> 0.125) -> ("x*y"=→"rad(NrTheta)_p":fxp<+/-,33,18>)
  }
  n233 = while "Atom_p" {
    shift-right: [w513] -> _
    shift-left: _ -> [w511]
    shift-right: [w512] -> _
    shift-left: _ -> [w510]
    shift-right: [w502] -> _
    shift-left: _ -> [w507]
    stop <- FALSE stop-if-true
    n234 = xnode "FPGA I/O Node"() -> ("Mod5/DI0"=w509:bool, "Mod5/DI1"=w508:bool)  [unwired: 2 in, 2 out]
    n235 = call "encoder_sub.vi"("A_pre"=w511, "B_pre"=w510, "Encoder Position_pre"=w507, "A input"=w509, "Encoder Position Reset"="Atom Reset", "B input"=w508) -> ("A"=w513:bool, "B"=w512:bool, "Encoder Position (Counts)"=w502:i32)  [unwired: 19 in]
    "Atom_Position_p" <- w502
    n236 = To Fixed-Point(number=w502) -> (fixed-point=w506:fxp<+/-,18,18>)  [unwired: 1 in]
    n237 = xnode ("High Throughput Multiply")("x"=w506, "y"=fxp<+/-,20,-5> -0.0009999871253967285) -> ("x*y"=w504:fxp<+/-,22,7>)
    "xp(mm)" <- w504
    n238 = Multiply(x=w504, y="kp") -> (x*y=→"fp":fxp<+/-,20,10>)
  }
  n239 = while "Db_d(M_avg method)" {
    shift-right: [w525] -> _
    shift-left: w24 -> [w528]
    tunnel: w26 -> [w526]
    shift-right: [w523] -> _
    shift-left: w25 -> [w521]
    shift-right: [w516] -> _
    shift-left: _ -> [w519]
    tunnel: w27 -> [w518]
    stop <- FALSE stop-if-true
    n240 = Index Array(array=w528, index=0) -> (element=w524:u32)
    n241 = Multiply(x=w526, y=w518) -> (x*y=w531:u32)
    n242 = Index Array(array=w521, index=0) -> (element=w520:i32)
    n243 = Add(x=w531, y=w524) -> (x+y=w530:u32)
    n244 = call "Tick Count5"() -> ("Tick Count(uSec)"=w527:u32)
    n245 = Greater Or Equal?(x=w527, y=w530) -> (x >= y?=w529:bool)
    n246 = case shown="True" w529 {
      tunnel: w528 -> [w536 w558]
      tunnel: w527 -> [_ w552]
      tunnel: w526 -> [_ w541]
      tunnel: [w536 w554] -> w525
      tunnel: w524 -> [_ w553]
      tunnel: w521 -> [w535 w542]
      tunnel: [w535 w540] -> w523
      tunnel: [w534 w539] -> w516
      tunnel: w520 -> [_ w537]
      tunnel: w519 -> [w534 _]
      frame False {
      }
      frame True {
        n247 = local read "Encoder Position_p"() -> (w546:i32)
        n248 = Subtract(x=w552, y=w553) -> (x-y=w551:u32)
        n249 = To Fixed-Point(number=w551) -> (fixed-point=w538:fxp<+,32,32>)  [unwired: 1 in]
        n250 = Insert Into Array(array=w558, index=w541, new element=w552) -> (w557:u32[])
        n251 = Insert Into Array(array=w542, index=w541, new element=w546) -> (w543:i32[])
        n252 = Subtract(x=w546, y=w537) -> (x-y=w547:i32)
        n253 = Multiply(x=w547, y=2500) -> (x*y=w549:i32)
        n254 = Delete From Array(array=w557, length=1, index=0) -> (array with subset deleted=w554:u32[])  [unwired: 1 out]
        n255 = Delete From Array(array=w543, length=1, index=0) -> (array with subset deleted=w540:i32[])  [unwired: 1 out]
        n256 = To Fixed-Point(number=w549) -> (fixed-point=w550:fxp<+/-,32,32>)  [unwired: 1 in]
        n257 = Divide(x=w550, y=w538) -> (x/y=w539:fxp<+/-,32,12>)
      }
    }
    "Dp_d(M_avg)" <- w516
    n258 = Multiply(x=w516, y=fxp<+/-,32,12> 3.1415929794311523 ("x")) -> (x*y=→"Omega_p(M_avg)":fxp<+/-,32,18>)
  }
  n259 = while "Db_d(M_avg method)" {
    shift-right: [w569] -> _
    shift-left: w23 -> [w572]
    tunnel: w21 -> [w570]
    shift-right: [w567] -> _
    shift-left: w22 -> [w565]
    shift-right: [w560] -> _
    shift-left: _ -> [w563]
    tunnel: w20 -> [w562]
    stop <- FALSE stop-if-true
    n260 = Index Array(array=w572, index=0) -> (element=w568:u32)
    n261 = Multiply(x=w570, y=w562) -> (x*y=w575:u32)
    n262 = Index Array(array=w565, index=0) -> (element=w564:i32)
    n263 = Add(x=w575, y=w568) -> (x+y=w574:u32)
    n264 = call "Tick Count13"() -> ("Tick Count(uSec)"=w571:u32)
    n265 = Greater Or Equal?(x=w571, y=w574) -> (x >= y?=w573:bool)
    n266 = case shown="True" w573 {
      tunnel: w572 -> [w580 w602]
      tunnel: w571 -> [_ w596]
      tunnel: w570 -> [_ w585]
      tunnel: [w580 w598] -> w569
      tunnel: w568 -> [_ w597]
      tunnel: w565 -> [w579 w586]
      tunnel: [w579 w584] -> w567
      tunnel: [w578 w583] -> w560
      tunnel: w564 -> [_ w581]
      tunnel: w563 -> [w578 _]
      frame False {
      }
      frame True {
        n267 = local read "Encoder Position_y"() -> (w590:i32)
        n268 = Subtract(x=w596, y=w597) -> (x-y=w595:u32)
        n269 = To Fixed-Point(number=w595) -> (fixed-point=w582:fxp<+,32,32>)  [unwired: 1 in]
        n270 = Insert Into Array(array=w602, index=w585, new element=w596) -> (w601:u32[])
        n271 = Insert Into Array(array=w586, index=w585, new element=w590) -> (w587:i32[])
        n272 = Subtract(x=w590, y=w581) -> (x-y=w591:i32)
        n273 = Multiply(x=w591, y=2500) -> (x*y=w593:i32)
        n274 = Delete From Array(array=w601, length=1, index=0) -> (array with subset deleted=w598:u32[])  [unwired: 1 out]
        n275 = Delete From Array(array=w587, length=1, index=0) -> (array with subset deleted=w584:i32[])  [unwired: 1 out]
        n276 = To Fixed-Point(number=w593) -> (fixed-point=w594:fxp<+/-,32,32>)  [unwired: 1 in]
        n277 = Divide(x=w594, y=w582) -> (x/y=w583:fxp<+/-,32,12>)
      }
    }
    "Dy_d(M_avg)" <- w560
    n278 = Multiply(x=w560, y=fxp<+/-,32,12> 3.1415929794311523 ("x")) -> (x*y=→"Omega_y(M_avg)":fxp<+/-,32,18>)
  }
  n279 = while "M_avg method" {
    shift-right: [w610] -> _
    shift-left: w31 -> [w613]
    shift-right: [w604] -> _
    shift-left: w28 -> [w607]
    tunnel: w30 -> [w611]
    shift-right: [w606] -> _
    shift-left: _ -> [w605]
    tunnel: w29 -> [w603]
    stop <- FALSE stop-if-true
    n280 = Index Array(array=w613, index=0) -> (element=w609:u32)
    n281 = Multiply(x=w611, y=w603) -> (x*y=w616:u32)
    n282 = Index Array(array=w607, index=0) -> (element=w608:i32)
    n283 = Add(x=w616, y=w609) -> (x+y=w615:u32)
    n284 = call "Tick Count7"() -> ("Tick Count(uSec)"=w612:u32)
    n285 = Greater Or Equal?(x=w612, y=w615) -> (x >= y?=w614:bool)
    n286 = case shown="True" w614 {
      tunnel: w613 -> [w622 w644]
      tunnel: w612 -> [_ w638]
      tunnel: w611 -> [_ w624]
      tunnel: [w622 w640] -> w610
      tunnel: w609 -> [_ w639]
      tunnel: w607 -> [w621 w635]
      tunnel: w608 -> [_ w631]
      tunnel: [w620 w626] -> w606
      tunnel: w605 -> [w620 _]
      tunnel: [w621 w625] -> w604
      frame False {
      }
      frame True {
        n287 = local read "Atom_Position_p"() -> (w632:i32)
        n288 = Subtract(x=w638, y=w639) -> (x-y=w637:u32)
        n289 = To Fixed-Point(number=w637) -> (fixed-point=w623:fxp<+,32,32>)  [unwired: 1 in]
        n290 = Insert Into Array(array=w644, index=w624, new element=w638) -> (w643:u32[])
        n291 = Insert Into Array(array=w635, index=w624, new element=w632) -> (w636:i32[])
        n292 = Subtract(x=w632, y=w631) -> (x-y=w630:i32)
        n293 = Multiply(x=w630, y=-1000) -> (x*y=w628:i32)
        n294 = Delete From Array(array=w643, length=1, index=0) -> (array with subset deleted=w640:u32[])  [unwired: 1 out]
        n295 = Delete From Array(array=w636, length=1, index=0) -> (array with subset deleted=w625:i32[])  [unwired: 1 out]
        n296 = To Fixed-Point(number=w628) -> (fixed-point=w627:fxp<+/-,32,32>)  [unwired: 1 in]
        n297 = Divide(x=w627, y=w623) -> (x/y=w626:fxp<+/-,25,10>)
      }
    }
    "xp_d(M_avg)" <- w606
  }
  n298 = while "M_avg method" {
    shift-right: [w652] -> _
    shift-left: w16 -> [w655]
    shift-right: [w646] -> _
    shift-left: w19 -> [w649]
    tunnel: w17 -> [w653]
    shift-right: [w648] -> _
    shift-left: _ -> [w647]
    tunnel: w18 -> [w645]
    stop <- FALSE stop-if-true
    n299 = Index Array(array=w655, index=0) -> (element=w651:u32)
    n300 = Multiply(x=w653, y=w645) -> (x*y=w658:u32)
    n301 = Index Array(array=w649, index=0) -> (element=w650:i32)
    n302 = Add(x=w658, y=w651) -> (x+y=w657:u32)
    n303 = call "Tick Count11"() -> ("Tick Count(uSec)"=w654:u32)
    n304 = Greater Or Equal?(x=w654, y=w657) -> (x >= y?=w656:bool)
    n305 = case shown="True" w656 {
      tunnel: w655 -> [w664 w686]
      tunnel: w654 -> [_ w680]
      tunnel: w653 -> [_ w666]
      tunnel: [w664 w682] -> w652
      tunnel: w651 -> [_ w681]
      tunnel: w649 -> [w663 w677]
      tunnel: w650 -> [_ w673]
      tunnel: [w662 w668] -> w648
      tunnel: w647 -> [w662 _]
      tunnel: [w663 w667] -> w646
      frame False {
      }
      frame True {
        n306 = local read "Atom_Position_y"() -> (w674:i32)
        n307 = Subtract(x=w680, y=w681) -> (x-y=w679:u32)
        n308 = To Fixed-Point(number=w679) -> (fixed-point=w665:fxp<+,32,32>)  [unwired: 1 in]
        n309 = Insert Into Array(array=w686, index=w666, new element=w680) -> (w685:u32[])
        n310 = Insert Into Array(array=w677, index=w666, new element=w674) -> (w678:i32[])
        n311 = Subtract(x=w674, y=w673) -> (x-y=w672:i32)
        n312 = Multiply(x=w672, y=-1000) -> (x*y=w670:i32)
        n313 = Delete From Array(array=w685, length=1, index=0) -> (array with subset deleted=w682:u32[])  [unwired: 1 out]
        n314 = Delete From Array(array=w678, length=1, index=0) -> (array with subset deleted=w667:i32[])  [unwired: 1 out]
        n315 = To Fixed-Point(number=w670) -> (fixed-point=w669:fxp<+/-,32,32>)  [unwired: 1 in]
        n316 = Divide(x=w669, y=w665) -> (x/y=w668:fxp<+/-,25,10>)
      }
    }
    "xy_d(M_avg)" <- w648
  }
  n317 = while "Encoder_y" {
    shift-right: [w689] -> _
    shift-left: _ -> [w700]
    shift-right: [w688] -> _
    shift-left: _ -> [w699]
    shift-right: [w692] -> _
    shift-left: _ -> [w698]
    stop <- FALSE stop-if-true
    n318 = local read "Encoder Reset"() -> (w687:bool)
    n319 = xnode "FPGA I/O Node"() -> ("Mod6/DI3"=w691:bool, "Mod6/DI4"=w690:bool)  [unwired: 2 in, 2 out]
    n320 = call "encoder_sub.vi"("A_pre"=w700, "B_pre"=w699, "Encoder Position_pre"=w698, "A input"=w691, "Encoder Position Reset"=w687, "B input"=w690) -> ("A"=w689:bool, "B"=w688:bool, "Encoder Position (Counts)"=w692:i32)  [unwired: 19 in]
    "Encoder Position_y" <- w692
    n321 = To Fixed-Point(number=w692) -> (fixed-point=w695:fxp<+/-,18,18>)  [unwired: 1 in]
    n322 = xnode ("High Throughput Multiply")("x"=w695, "y"=fxp<+/-,15,-7> 0.0012500286102294922) -> ("x*y"=→"Dy(mm)":fxp<+/-,22,7>)
    n323 = xnode ("High Throughput Multiply")("x"=w695, "y"=fxp<+,24,0> 0.125) -> ("x*y"=→"rad(NrTheta)_y":fxp<+/-,33,18>)
  }
  n324 = while "Atom_y" {
    shift-right: [w715] -> _
    shift-left: _ -> [w713]
    shift-right: [w714] -> _
    shift-left: _ -> [w712]
    shift-right: [w705] -> _
    shift-left: _ -> [w709]
    stop <- FALSE stop-if-true
    n325 = local read "Atom Reset"() -> (w703:bool)
    n326 = xnode "FPGA I/O Node"() -> ("Mod6/DI0"=w711:bool, "Mod6/DI1"=w710:bool)  [unwired: 2 in, 2 out]
    n327 = call "encoder_sub.vi"("A_pre"=w713, "B_pre"=w712, "Encoder Position_pre"=w709, "A input"=w711, "Encoder Position Reset"=w703, "B input"=w710) -> ("A"=w715:bool, "B"=w714:bool, "Encoder Position (Counts)"=w705:i32)  [unwired: 19 in]
    "Atom_Position_y" <- w705
    n328 = To Fixed-Point(number=w705) -> (fixed-point=w708:fxp<+/-,18,18>)  [unwired: 1 in]
    n329 = xnode ("High Throughput Multiply")("x"=w708, "y"=fxp<+/-,20,-5> -0.0009999871253967285) -> ("x*y"=w706:fxp<+/-,22,7>)
    "xy(mm)" <- w706
    n330 = Multiply(x=w706, y="ky") -> (x*y=→"fy":fxp<+/-,20,10>)
  }
  n331 = while "Velocity estimation methods" {
    stop <- FALSE stop-if-true
    n332 = case shown="0, Default" "Encoder (P/Y)\nVelocity Method" {
      tunnel: [w739] -> w728
      tunnel: [w738] -> w727
      tunnel: [w737] -> w726
      tunnel: [w736] -> w725
      frame 0, Default {
        n333 = local read "Omega_p(M_avg)"() -> (w737:fxp<+/-,32,18>)
        n334 = local read "Dy_d(M_avg)"() -> (w738:fxp<+/-,32,12>)
        n335 = local read "Omega_y(M_avg)"() -> (w739:fxp<+/-,32,18>)
        n336 = local read "Dp_d(M_avg)"() -> (w736:fxp<+/-,32,12>)
      }
    }
    "Dp_d(mm/s)" <- w725
    "Omega_p(rad/s)" <- w726
    "Dy_d(mm/s)" <- w727
    "Omega_y(rad/s)" <- w728
    n337 = case shown="0, Default" "Encoder b\nVelocity method" {
      tunnel: [w735] -> w723
      tunnel: [w734] -> w724
      frame 0, Default {
        n338 = local read "Db_d(M_avg method)"() -> (w735:fxp<+/-,32,12>)
        n339 = local read "Omega_b(M_avg)"() -> (w734:fxp<+/-,32,18>)
      }
    }
    "Db_d(mm/s)" <- w723
    "Omega_b(rad/s)" <- w724
    n340 = case shown="0, Default" "ATOM b\nVelocity method" {
      tunnel: [w733] -> w721
      frame 0, Default {
        n341 = local read "xb_d(M_avg method)"() -> (w733:fxp<+/-,25,10>)
      }
    }
    "xb_d(mm/s)" <- w721
    n342 = case shown="0, Default" "ATOM (P/Y)\nVelocity Method" {
      tunnel: [w732] -> w718
      tunnel: [w731] -> w719
      frame 0, Default {
        n343 = local read "xp_d(M_avg)"() -> (w732:fxp<+/-,25,10>)
        n344 = local read "xy_d(M_avg)"() -> (w731:fxp<+/-,25,10>)
      }
    }
    "xp_d(mm/s)" <- w718
    "xy_d(mm/s)" <- w719
  }
  n345 = while "Switch case" {
    stop <- FALSE stop-if-true
    n346 = case shown="2" "CASE (py)" {
      frame 0, Default {
        n347 = local write "Forward/Backward (py)"(FALSE ("Forward/Backward")) -> ()
        n348 = local write "Bvp"(fxp<+,10,3> 0.0 ("Bvp")) -> ()
        n349 = local write "Kvp"(fxp<+,15,8> 0.0 ("Kvp")) -> ()
        n350 = local write "Bvy"(fxp<+,10,3> 0.0 ("Bvy")) -> ()
        n351 = local write "Kvy"(fxp<+,15,8> 0.0 ("Kvp")) -> ()
      }
      frame 1 {
        n352 = local write "Forward/Backward (py)"(TRUE ("Forward/Backward")) -> ()
      }
      frame 2 {
        w762 = i16 0 items=["Step", "Sin"] ("Step / Sin (py)")
        n353 = local write "Forward/Backward (py)"(TRUE ("Forward/Backward")) -> ()
        n354 = local write "Step / Sin (py)"(w762) -> ()
        n355 = local write "Dpr"(fxp<+/-,22,8> 0.0 ("Dpr")) -> ()
        n356 = local write "Dyr"(fxp<+/-,22,8> 0.0 ("Dyr")) -> ()
      }
    }
    n357 = case shown="0, Default" "Step / Sin (py)" {
      frame 0, Default {
        n358 = local write "Step/Sin Dpy"(FALSE ("Inv./Pos.")) -> ()
      }
      frame 1 {
        n359 = local write "Step/Sin Dpy"(TRUE ("Inv./Pos.")) -> ()
      }
    }
    n360 = case shown="0, Default" "Sin/Step (b)" {
      frame 0, Default {
        n361 = local write "Step/Sin Db"(FALSE ("Inv./Pos.")) -> ()
      }
      frame 1 {
        n362 = local write "Step/Sin Db"(TRUE ("Inv./Pos.")) -> ()
      }
    }
    n363 = case shown="2" "CASE (b)" {
      frame 0, Default {
        n364 = local write "Forward/Backward (b)"(FALSE ("Forward/Backward")) -> ()
        n365 = local write "Kvb"(fxp<+,15,8> 0.0 ("Kvp")) -> ()
        n366 = local write "Bvb"(fxp<+,10,3> 0.0 ("Bvp")) -> ()
      }
      frame 1 {
        n367 = local write "Forward/Backward (b)"(TRUE ("Forward/Backward")) -> ()
      }
      frame 2 {
        w749 = i16 0 items=["Step", "Sin"] ("Sin/Step (b)")
        n368 = local write "Forward/Backward (b)"(TRUE ("Forward/Backward")) -> ()
        n369 = local write "Sin/Step (b)"(w749) -> ()
        n370 = local write "Dbr"(fxp<+/-,22,8> 0.0 ("Dpr")) -> ()
      }
    }
  }
  n371 = while "FIFO_p" {
    stop <- FALSE stop-if-true
    n372 = flat-sequence {
      tunnel: [w769] -> w766
      tunnel: w766 -> [w798]
      frame #0 {
        n373 = call "Loop Timer"("Count(uSec)"=u32 1000 ("Loop Period (usec)")) -> ()  [unwired: 1 out]
      }
      frame #1 {
        n374 = case shown="2" "FIFO" {
          tunnel: [w779 w788 w789] -> w769
          frame 0, Default {
            n375 = local read "Dp(mm)"() -> (w778:fxp<+/-,22,7>)
            n376 = local read "xp(mm)"() -> (w777:fxp<+/-,22,7>)
            n377 = local read "Db(mm)"() -> (w776:fxp<+/-,22,7>)
            n378 = local read "xb(mm)"() -> (w775:fxp<+/-,22,7>)
            n379 = local read "Dy(mm)"() -> (w774:fxp<+/-,22,7>)
            n380 = local read "xy(mm)"() -> (w773:fxp<+/-,22,7>)
            n381 = local read "fp_tilde"() -> (w772:fxp<+/-,21,11>)
            n382 = local read "fpt_i"() -> (w771:fxp<+/-,32,9>)
            n383 = Build Array(w778, w777, w776, w775, w774, w773, w772, w771) -> (w779:fxp<+/-,34,11>[])
          }
          frame 1 {
            n384 = local read "fp_tilde"() -> (w781:fxp<+/-,21,11>)
            n385 = local read "fpt_i"() -> (w780:fxp<+/-,32,9>)
            n386 = local read "Dpr_sin/cos"() -> (w787:fxp<+/-,24,10>)
            n387 = local read "Dp(mm)"() -> (w786:fxp<+/-,22,7>)
            n388 = local read "xp(mm)"() -> (w785:fxp<+/-,22,7>)
            n389 = local read "Dyr_sin/cos"() -> (w784:fxp<+/-,24,10>)
            n390 = local read "Dy(mm)"() -> (w783:fxp<+/-,22,7>)
            n391 = local read "xy(mm)"() -> (w782:fxp<+/-,22,7>)
            n392 = Build Array(w787, w786, w785, w784, w783, w782, w780, w781) -> (w788:fxp<+/-,34,11>[])
          }
          frame 2 {
            n393 = local read "Dabr_sin/cos"() -> (w794:fxp<+/-,22,8>)
            n394 = local read "Db(mm)"() -> (w793:fxp<+/-,22,7>)
            n395 = local read "xb(mm)"() -> (w792:fxp<+/-,22,7>)
            n396 = local read "Dpr_sin/cos"() -> (w797:fxp<+/-,24,10>)
            n397 = local read "Dp(mm)"() -> (w796:fxp<+/-,22,7>)
            n398 = local read "xp(mm)"() -> (w795:fxp<+/-,22,7>)
            n399 = local read "fpt_i"() -> (w790:fxp<+/-,32,9>)
            n400 = local read "fp_tilde"() -> (w791:fxp<+/-,21,11>)
            n401 = Build Array(w797, w796, w795, w794, w793, w792, w790, w791) -> (w789:fxp<+/-,34,11>[])
          }
        }
      }
      frame #2 {
        n402 = xnode ("FIFO Method Node")("Element"=w798, "Timeout"=0) -> ()  [unwired: 1 in, 2 out]
      }
    }
  }
  n403 = while "cycle_stop & Impact protection pyb" {
    stop <- FALSE stop-if-true
    n404 = local read "Forward/Backward (b)"() -> (w816:bool)
    n405 = local read "Forward/Backward (py)"() -> (w817:bool)
    n406 = local read "Stop Motor_b"() -> (w813:bool)
    n407 = local read "Stop Motor"() -> (w820:bool)
    n408 = local read "fy"() -> (w804:fxp<+/-,20,10>)
    n409 = local read "fp"() -> (w801:fxp<+/-,20,10>)
    n410 = local read "fb"() -> (w812:fxp<+/-,20,10>)
    n411 = Not(x=w820) -> (.not. x?=w818:bool)
    n412 = Not(x=w813) -> (.not. x?=w815:bool)
    n413 = Absolute Value(x=w801) -> (abs(x)=w802:fxp<+,20,10>)
    n414 = Absolute Value(x=w804) -> (abs(x)=w803:fxp<+,20,10>)
    n415 = Not And(1:w818, 2:w817) -> (0:w819:bool)
    n416 = Not And(1:w815, 2:w816) -> (0:w814:bool)
    n417 = Absolute Value(x=w812) -> (abs(x)=w811:fxp<+,20,10>)
    n418 = Greater?(x=w802, y="fpy_Impact") -> (0:w806:bool)
    n419 = Greater?(x=w803, y="fpy_Impact") -> (0:w805:bool)
    n420 = case shown="False" w819 {
      frame False {
        n421 = local read "Sin wave time (s)"() -> (w832:fxp<+,64,32>)
        n422 = Greater?(x=w832, y="time stop py") -> (0:w830:bool)
        n423 = local write "Stop Motor"(w830) -> ()
      }
      frame True {
      }
    }
    n424 = case shown="False" w814 {
      frame False {
        n425 = local read "Sin wave time (s) b"() -> (w829:fxp<+,64,32>)
        n426 = Greater?(x=w829, y="time stop b") -> (0:w827:bool)
        n427 = local write "Stop Motor_b"(w827) -> ()
      }
      frame True {
      }
    }
    n428 = Greater?(x=w811, y="fb_lmpact") -> (0:w809:bool)
    n429 = Or(x=w805, y=w806) -> (x .or. y?=w807:bool)
    n430 = case shown="True" w809 {
      frame False {
      }
      frame True {
        n431 = local write "Stop Motor_b"(TRUE ("Stop Motor_b")) -> ()
        n432 = local write "Stop Motor"(TRUE ("Stop Motor_b")) -> ()
      }
    }
    n433 = case shown="True" "Start_two" {
      frame False {
      }
      frame True {
        w822 = FALSE ("Stop Motor_b")
        n434 = local write "Stop Motor"(w822) -> ()
        n435 = local write "Stop Motor_b"(w822) -> ()
      }
    }
    n436 = case shown="True" w807 {
      frame False {
      }
      frame True {
        n437 = local write "Stop Motor_b"(TRUE ("Stop Motor_b")) -> ()
        n438 = local write "Stop Motor"(TRUE ("Stop Motor_b")) -> ()
      }
    }
  }
  n439 = while "Derivative_pyb" {
    stop <- FALSE stop-if-true
    n440 = flat-sequence {
      tunnel: [w845] -> w838
      tunnel: [w844] -> w837
      tunnel: [w843] -> w836
      tunnel: [w842] -> w835
      tunnel: [w841] -> w834
      tunnel: [w840] -> w833
      tunnel: w838 -> [w889]
      tunnel: w837 -> [w888]
      tunnel: w836 -> [w887]
      tunnel: w835 -> [w886]
      tunnel: w834 -> [w885]
      tunnel: w833 -> [w884]
      frame #0 {
        n441 = local read "Db_d(mm/s)"() -> (w850:fxp<+/-,32,12>)
        n442 = local read "xb_d(mm/s)"() -> (w848:fxp<+/-,25,10>)
        n443 = local read "Dabr_d"() -> (w851:fxp<+/-,33,10>)
        n444 = local read "Dabr_dd"() -> (w852:fxp<+/-,34,12>)
        n445 = local read "Db_dd"() -> (w853:fxp<+/-,25,15>)
        n446 = local read "xb_dd"() -> (w855:fxp<+/-,25,15>)
        n447 = local read "Dpr_d"() -> (w880:fxp<+/-,35,12>)
        n448 = local read "Dp_d(mm/s)"() -> (w881:fxp<+/-,32,12>)
        n449 = local read "xp_d(mm/s)"() -> (w883:fxp<+/-,25,10>)
        n450 = local read "Dpr_dd"() -> (w879:fxp<+/-,36,14>)
        n451 = local read "Dp_dd"() -> (w878:fxp<+/-,25,15>)
        n452 = local read "xp_dd"() -> (w860:fxp<+/-,25,15>)
        n453 = local read "Dyr_d"() -> (w864:fxp<+/-,35,12>)
        n454 = local read "Dyr_dd"() -> (w865:fxp<+/-,36,14>)
        n455 = local read "Dy_dd"() -> (w866:fxp<+/-,25,15>)
        n456 = local read "xy_dd"() -> (w868:fxp<+/-,25,15>)
        n457 = local read "Dy_d(mm/s)"() -> (w863:fxp<+/-,32,12>)
        n458 = local read "xy_d(mm/s)"() -> (w861:fxp<+/-,25,10>)
        n459 = local read "Stop Motor_b"() -> (w858:bool)
        n460 = local read "Stop Motor"() -> (w859:bool)
        n461 = Subtract(x=w864, y=w863) -> (x-y=w862:fxp<+/-,33,10>)
        n462 = Subtract(x=w865, y=w866) -> (x-y=w867:fxp<+/-,38,16>)
        n463 = Subtract(x=w880, y=w881) -> (x-y=w882:fxp<+/-,33,10>)
        n464 = Subtract(x=w879, y=w878) -> (x-y=w877:fxp<+/-,38,16>)
        n465 = Subtract(x=w851, y=w850) -> (x-y=w849:fxp<+/-,33,10>)
        n466 = Subtract(x=w852, y=w853) -> (x-y=w854:fxp<+/-,38,16>)
        n467 = Add(x=w867, y=w868) -> (x+y=w871:fxp<+/-,34,12>)
        n468 = Add(x=w877, y=w860) -> (x+y=w874:fxp<+/-,34,12>)
        n469 = Add(x=w854, y=w855) -> (x+y=w857:fxp<+/-,34,12>)
        n470 = Add(x=w862, y=w861) -> (x+y=w869:fxp<+/-,33,10>)
        n471 = Add(x=w882, y=w883) -> (x+y=w876:fxp<+/-,33,10>)
        n472 = Add(x=w849, y=w848) -> (x+y=w856:fxp<+/-,33,10>)
        n473 = Select(t=fxp<+/-,33,10> 0.0, s=w859, f=w869) -> (s? t:f=w841:fxp<+/-,33,10>)
        "Dy_ed" <- w841
        n474 = Select(t=fxp<+/-,33,10> 0.0, s=w859, f=w876) -> (s? t:f=w843:fxp<+/-,33,10>)
        "Dp_ed" <- w843
        n475 = Select(t=fxp<+/-,34,12> 0.0, s=w859, f=w871) -> (s? t:f=w840:fxp<+/-,34,12>)
        "Dy_edd" <- w840
        n476 = Select(t=fxp<+/-,34,12> 0.0, s=w859, f=w874) -> (s? t:f=w842:fxp<+/-,34,12>)
        "Dp_edd" <- w842
        n477 = Select(t=fxp<+/-,33,10> 0.0, s=w858, f=w856) -> (s? t:f=w845:fxp<+/-,33,10>)
        "Dab_ed" <- w845
        n478 = Select(t=fxp<+/-,34,12> 0.0, s=w858, f=w857) -> (s? t:f=w844:fxp<+/-,34,12>)
        "Dab_edd" <- w844
      }
      frame #1 {
        n479 = local read "xp_d(mm/s)"() -> (w913:fxp<+/-,25,10>)
        n480 = local read "xy_d(mm/s)"() -> (w909:fxp<+/-,25,10>)
        n481 = local read "xb_d(mm/s)"() -> (w922:fxp<+/-,25,10>)
        n482 = local read "Bvp"() -> (w899:fxp<+,10,3>)
        n483 = local read "Kvp"() -> (w898:fxp<+,15,8>)
        n484 = local read "Bvy"() -> (w904:fxp<+,10,3>)
        n485 = local read "Kvb"() -> (w918:fxp<+,15,8>)
        n486 = local read "Kvy"() -> (w905:fxp<+,15,8>)
        n487 = local read "Bvb"() -> (w917:fxp<+,15,8>)
        n488 = local read "Stop Motor_b"() -> (w916:bool)
        n489 = Multiply(x=w887, y=w898) -> (x*y=w897:fxp<+/-,48,18>)
        n490 = Multiply(x=w886, y=w899) -> (x*y=w896:fxp<+/-,44,15>)
        n491 = Multiply(x=w885, y=w905) -> (x*y=w906:fxp<+/-,48,18>)
        n492 = Multiply(x=w884, y=w904) -> (x*y=w907:fxp<+/-,44,15>)
        n493 = local read "kp"() -> (w894:fxp<+,15,8>)
        n494 = Multiply(x=w889, y=w918) -> (x*y=w919:fxp<+/-,48,18>)
        n495 = Multiply(x=w888, y=w917) -> (x*y=w920:fxp<+/-,49,20>)
        n496 = local read "Stop Motor"() -> (w912:bool)
        n497 = local read "ky"() -> (w910:fxp<+,15,8>)
        n498 = local read "kb"() -> (w923:fxp<+,15,8>)
        n499 = Add(x=w897, y=w896) -> (x+y=w895:fxp<+/-,49,19>)
        n500 = Add(x=w906, y=w907) -> (x+y=w908:fxp<+/-,49,19>)
        n501 = Add(x=w919, y=w920) -> (x+y=w921:fxp<+/-,50,20>)
        n502 = Multiply(x=w894, y=w913) -> (x*y=w893:fxp<+/-,35,12>)
        n503 = Multiply(x=w910, y=w909) -> (x*y=w911:fxp<+/-,35,12>)
        n504 = Multiply(x=w923, y=w922) -> (x*y=w924:fxp<+/-,35,12>)
        n505 = Subtract(x=w895, y=w893) -> (x-y=w900:fxp<+/-,25,15>)
        n506 = Subtract(x=w908, y=w911) -> (x-y=w903:fxp<+/-,25,15>)
        n507 = Subtract(x=w921, y=w924) -> (x-y=w915:fxp<+/-,25,15>)
        n508 = Select(t=fxp<+/-,25,15> 0.0, s=w912, f=w900) -> (s? t:f=→"fpt_d":fxp<+/-,25,15>)
        n509 = Select(t=fxp<+/-,25,15> 0.0, s=w912, f=w903) -> (s? t:f=→"fyt_d":fxp<+/-,25,15>)
        n510 = Select(t=fxp<+/-,25,15> 0.0, s=w916, f=w915) -> (s? t:f=→"fbt_d":fxp<+/-,25,15>)
      }
    }
  }
  n511 = local write "Atom Reset"(w1) -> ()
  n512 = local write "Encoder Reset"(w1) -> ()
  n513 = local write "Coe Ini"(w1) -> ()
  n514 = local write "dFb_PID_add"(w1) -> ()
  n515 = local write "Stop Motor_b"(w5) -> ()
  n516 = local write "Stop Motor"(w5) -> ()
  n517 = local write "Encoder Reset_b"(w2) -> ()
  n518 = local write "Atom Reset_b"(w2) -> ()
  n519 = local write "Dpy_d_M_avg_Tc (uSec)"(u32 1000 ("M_avg_Tc (uSec)")) -> ()
  n520 = local write "xpy_d_M_avg_Tc (uSec)"(u32 40 ("M_avg_Tc (uSec)")) -> ()
  n521 = local write "Db_d_M_avg_Tc (uSec)"(u32 1000 ("M_avg_Tc (uSec)")) -> ()
  n522 = local write "xb_d_M_avg_Tc (uSec)"(u32 40 ("M_avg_Tc (uSec)")) -> ()
  n523 = local write "Start_two"(w1) -> ()
  n524 = while "Intergral and  derivative" {
    shift-right: [w1028] -> _
    shift-left: _ -> [w1029]
    shift-right: [w1015] -> _
    shift-left: _ -> [w1034]
    shift-right: [w1024] -> _
    shift-left: _ -> [w1022]
    shift-right: [w1008] -> _
    shift-left: _ -> [w1009]
    shift-right: [w1007] -> _
    shift-left: _ -> [w1006]
    shift-right: [w972] -> _
    shift-left: _ -> [w971]
    shift-right: [w970] -> _
    shift-left: _ -> [w969]
    shift-right: [w968] -> _
    shift-left: _ -> [w967]
    shift-right: [w966] -> _
    shift-left: _ -> [w965]
    shift-right: [w964] -> _
    shift-left: _ -> [w963]
    shift-right: [w935] -> _
    shift-left: _ -> [w934]
    shift-right: [w933] -> _
    shift-left: _ -> [w932]
    shift-right: [w931] -> _
    shift-left: _ -> [w930]
    shift-right: [w929] -> _
    shift-left: _ -> [w928]
    shift-right: [w927] -> _
    shift-left: _ -> [w926]
    stop <- FALSE stop-if-true
    n525 = local read "fy_tolerance"() -> (w940:fxp<+,32,9>)
    n526 = local read "scaled coe_Dpy_dd"() -> (w961:i32[])
    n527 = local read "fp_tilde"() -> (w980:fxp<+/-,21,11>)
    n528 = local read "fy_tilde"() -> (w942:fxp<+/-,21,11>)
    n529 = local read "fb_tilde"() -> (w1030:fxp<+/-,21,11>)
    n530 = local read "scaled coe_xpy_dd"() -> (w962:i32[])
    n531 = local read "Dp_d(mm/s)"() -> (w966:fxp<+/-,32,12>)
    n532 = local read "Dy_d(mm/s)"() -> (w929:fxp<+/-,32,12>)
    n533 = local read "fp_tolerance"() -> (w978:fxp<+,32,9>)
    n534 = local read "Db_d(mm/s)"() -> (w1008:fxp<+/-,32,12>)
    n535 = local read "xp_d(mm/s)"() -> (w964:fxp<+/-,25,10>)
    n536 = local read "fb_tolerance"() -> (w1032:fxp<+,32,9>)
    n537 = local read "xy_d(mm/s)"() -> (w927:fxp<+/-,25,10>)
    n538 = local read "xb_d(mm/s)"() -> (w1007:fxp<+/-,25,10>)
    n539 = local read "scaled coe_dFpy_PID"() -> (w960:i32[])
    n540 = local read "Fp_PID"() -> (w968:fxp<+/-,21,11>)
    n541 = local read "Fy_PID"() -> (w931:fxp<+/-,21,11>)
    n542 = local read "Fb_PID"() -> (w1024:fxp<+/-,21,11>)
    n543 = Absolute Value(x=w980) -> (abs(x)=w977:fxp<+,21,11>)
    n544 = Absolute Value(x=w942) -> (abs(x)=w939:fxp<+,21,11>)
    n545 = Absolute Value(x=w1030) -> (abs(x)=w1033:fxp<+,21,11>)
    n546 = local read "Stop Motor_b"() -> (w1036:bool)
    n547 = Greater?(x=w977, y=w978) -> (0:w979:bool)
    n548 = Greater?(x=w939, y=w940) -> (0:w941:bool)
    n549 = Greater?(x=w1033, y=w1032) -> (0:w1031:bool)
    n550 = Subtract(x=w966, y=w965) -> (x-y=w994:fxp<+/-,33,13>)
    n551 = Subtract(x=w929, y=w928) -> (x-y=w954:fxp<+/-,33,13>)
    n552 = Subtract(x=w964, y=w963) -> (x-y=w997:fxp<+/-,26,11>)
    n553 = Subtract(x=w927, y=w926) -> (x-y=w957:fxp<+/-,26,11>)
    n554 = Subtract(x=w1008, y=w1009) -> (x-y=w1011:fxp<+/-,33,13>)
    n555 = Subtract(x=w1007, y=w1006) -> (x-y=w1004:fxp<+/-,26,11>)
    n556 = Subtract(x=w968, y=w967) -> (x-y=w984:fxp<+/-,22,12>)
    n557 = Subtract(x=w931, y=w930) -> (x-y=w946:fxp<+/-,22,12>)
    n558 = Subtract(x=w1024, y=w1022) -> (x-y=w1023:fxp<+/-,22,12>)
    n559 = local read "Stop Motor"() -> (w975:bool)
    n560 = local read "Stop Motor"() -> (w937:bool)
    n561 = Select(t=w980, s=w979, f=fxp<+/-,21,11> 0.0) -> (s? t:f=w972:fxp<+/-,21,11>)
    n562 = Select(t=w942, s=w941, f=fxp<+/-,21,11> 0.0) -> (s? t:f=w935:fxp<+/-,21,11>)
    n563 = Select(t=w1030, s=w1031, f=fxp<+/-,21,11> 0.0) -> (s? t:f=w1028:fxp<+/-,21,11>)
    n564 = Add(x=w972, y=w971) -> (x+y=w973:fxp<+/-,22,12>)
    n565 = Add(x=w935, y=w934) -> (x+y=w925:fxp<+/-,22,12>)
    n566 = Add(x=w1028, y=w1029) -> (x+y=w1038:fxp<+/-,22,12>)
    n567 = Multiply(x=w994, y=fxp<+,10,10> 1000.0) -> (x*y=w993:fxp<+/-,25,15>)
    n568 = Multiply(x=w954, y=fxp<+,10,10> 1000.0) -> (x*y=w953:fxp<+/-,25,15>)
    n569 = Multiply(x=w997, y=fxp<+,10,10> 1000.0) -> (x*y=w998:fxp<+/-,25,15>)
    n570 = Multiply(x=w957, y=fxp<+,10,10> 1000.0) -> (x*y=w958:fxp<+/-,25,15>)
    n571 = Multiply(x=w1011, y=fxp<+,10,10> 1000.0) -> (x*y=w1012:fxp<+/-,25,15>)
    n572 = Multiply(x=w1004, y=fxp<+,10,10> 1000.0) -> (x*y=w1003:fxp<+/-,25,15>)
    n573 = Multiply(x=w984, y=fxp<+,10,10> 1000.0) -> (x*y=w985:fxp<+/-,25,15>)
    n574 = Multiply(x=w946, y=fxp<+,10,10> 1000.0) -> (x*y=w947:fxp<+/-,25,15>)
    n575 = Multiply(x=w1023, y=fxp<+,10,10> 1000.0) -> (x*y=w1021:fxp<+/-,25,15>)
    n576 = Multiply(x=w973, y=fxp<+/-,9,-9> 0.000499725341796875) -> (x*y=w976:fxp<+/-,31,3>)
    n577 = Multiply(x=w925, y=fxp<+/-,9,-9> 0.000499725341796875) -> (x*y=w938:fxp<+/-,31,3>)
    n578 = Multiply(x=w1038, y=fxp<+/-,9,-9> 0.000499725341796875) -> (x*y=w1035:fxp<+/-,31,3>)
    n579 = Add(x=w976, y=w969) -> (x+y=w990:fxp<+/-,30,7>)
    n580 = Add(x=w938, y=w932) -> (x+y=w951:fxp<+/-,30,7>)
    n581 = Add(x=w1035, y=w1034) -> (x+y=w1016:fxp<+/-,30,7>)
    n582 = Select(t=fxp<+/-,2,2> 0.0, s=w975, f=fxp<+/-,2,2> 1.0) -> (s? t:f=w989:fxp<+/-,2,2>)
    n583 = Select(t=fxp<+/-,2,2> 0.0, s=w937, f=fxp<+/-,2,2> 1.0) -> (s? t:f=w950:fxp<+/-,2,2>)
    n584 = Select(t=fxp<+/-,2,2> 0.0, s=w1036, f=fxp<+/-,2,2> 1.0) -> (s? t:f=w1017:fxp<+/-,2,2>)
    n585 = xnode "Butterworth Filter"("input data"=w993, "scaled coefficients"="scaled coe_Dpy_dd") -> ("output data"=→"Dp_dd":fxp<+/-,25,15>)  [unwired: 1 in]
    n586 = xnode "Butterworth Filter"("input data"=w953, "scaled coefficients"=w961) -> ("output data"=→"Dy_dd":fxp<+/-,25,15>)  [unwired: 1 in]
    n587 = xnode "Butterworth Filter"("input data"=w998, "scaled coefficients"="scaled coe_xpy_dd") -> ("output data"=→"xp_dd":fxp<+/-,25,15>)  [unwired: 1 in]
    n588 = xnode "Butterworth Filter"("input data"=w958, "scaled coefficients"=w962) -> ("output data"=→"xy_dd":fxp<+/-,25,15>)  [unwired: 1 in]
    n589 = xnode "Butterworth Filter"("input data"=w1012, "scaled coefficients"="scaled coe_Db_dd") -> ("output data"=→"Db_dd":fxp<+/-,25,15>)  [unwired: 1 in]
    n590 = xnode "Butterworth Filter"("input data"=w1003, "scaled coefficients"="scaled coe_xb_dd") -> ("output data"=→"xb_dd":fxp<+/-,25,15>)  [unwired: 1 in]
    n591 = xnode "Butterworth Filter"("input data"=w985, "scaled coefficients"="scaled coe_dFpy_PID") -> ("output data"=→"dFp_PID":fxp<+/-,25,15>)  [unwired: 1 in]
    n592 = xnode "Butterworth Filter"("input data"=w947, "scaled coefficients"=w960) -> ("output data"=→"dFy_PID":fxp<+/-,25,15>)  [unwired: 1 in]
    n593 = xnode "Butterworth Filter"("input data"=w1021, "scaled coefficients"="scaled coe_dFb_PID") -> ("output data"=→"dFb_PID":fxp<+/-,25,15>)  [unwired: 1 in]
    n594 = Multiply(x=w990, y=w989) -> (x*y=w970:fxp<+/-,32,9>)
    "fpt_i" <- w970
    n595 = Multiply(x=w951, y=w950) -> (x*y=w933:fxp<+/-,32,9>)
    "fyt_i" <- w933
    n596 = Multiply(x=w1016, y=w1017) -> (x*y=w1015:fxp<+/-,32,9>)
    "fbt_i" <- w1015
    n597 = call "Wait8"("Count(uSec)"=u32 1000 ("Count(mSec)")) -> ()  [unwired: 1 out]
  }
  n598 = while "Time reset" {
    shift-right: [w1123] -> _
    shift-left: _ -> [w1124]
    shift-right: [w1115] -> _
    shift-left: _ -> [w1117]
    stop <- FALSE stop-if-true
    n599 = call "Tick Count"() -> ("Tick Count(uSec)"=w1123:u32)
    n600 = local read "Stop Motor"() -> (w1120:bool)
    n601 = Subtract(x=w1123, y=w1124) -> (x-y=w1119:u32)
    n602 = Add(x=w1117, y=w1119) -> (x+y=w1118:u32)
    n603 = Select(t=u32 0, s=w1120, f=w1118) -> (s? t:f=w1115:u32)
    n604 = To Fixed-Point(number=w1115) -> (fixed-point=w1113:fxp<+,64,32>)  [unwired: 1 in]
    n605 = Multiply(x=fxp<+,20,-18> 1.0000003385357559e-06 ("y"), y=w1113) -> (x*y=→"Sin wave time (s)":fxp<+,64,32>)
  }
  n606 = while "Time reset" {
    shift-right: [w1135] -> _
    shift-left: _ -> [w1136]
    shift-right: [w1127] -> _
    shift-left: _ -> [w1129]
    stop <- FALSE stop-if-true
    n607 = local read "Stop Motor_b"() -> (w1132:bool)
    n608 = call "Tick Count15"() -> ("Tick Count(uSec)"=w1135:u32)
    n609 = Subtract(x=w1135, y=w1136) -> (x-y=w1131:u32)
    n610 = Add(x=w1129, y=w1131) -> (x+y=w1130:u32)
    n611 = Select(t=u32 0, s=w1132, f=w1130) -> (s? t:f=w1127:u32)
    n612 = To Fixed-Point(number=w1127) -> (fixed-point=w1125:fxp<+,64,32>)  [unwired: 1 in]
    n613 = Multiply(x=fxp<+,20,-18> 1.0000003385357559e-06 ("y"), y=w1125) -> (x*y=→"Sin wave time (s) b":fxp<+,64,32>)
  }
  n614 = while "Coe_in" {
    stop <- FALSE stop-if-true
    n615 = case shown="True" "Coe Ini" {
      frame False {
      }
      frame True {
        w1140 = fxp<+,15,8> 58.640625 ("kb")
        w1147 = fxp<+,32,9> 0.20000004768371582 ("fp_tolerance")
        w1139 = fxp<+,15,8> 23.5390625 ("kp t")
        n616 = local write "Kpy"(fxp<+,11,7> 40.0 ("Kpb")) -> ()
        n617 = local write "Kiy"(fxp<+,27,10> 0.0 ("Kib")) -> ()
        n618 = local write "Kdy"(fxp<+,26,2> 0.0 ("Kdb")) -> ()
        n619 = local write "fpy_Impact"(fxp<+,10,5> 30.0 ("fb_limit")) -> ()
        n620 = local write "Kpp"(fxp<+,11,7> 60.0 ("Kpb")) -> ()
        n621 = local write "Kip"(fxp<+,27,10> 0.0 ("Kib")) -> ()
        n622 = local write "Kdp"(fxp<+,26,2> 0.0 ("Kdb")) -> ()
        n623 = local write "ky"(w1139) -> ()
        n624 = local write "kp"(w1139) -> ()
        n625 = local write "fp_tolerance"(w1147) -> ()
        n626 = local write "fy_tolerance"(w1147) -> ()
        n627 = local write "Kdb"(fxp<+,26,2> 0.5 ("Kdb")) -> ()
        n628 = local write "Kpb"(fxp<+,11,7> 40.0 ("Kpb")) -> ()
        n629 = local write "Kib"(fxp<+,27,10> 20.0 ("Kib")) -> ()
        n630 = local write "fb_lmpact"(fxp<+,10,5> 30.0 ("fb_limit")) -> ()
        n631 = Multiply(x=w1140, y=fxp<+,17,1> 0.0200042724609375 ("kb")) -> (x*y=w1146:fxp<+,32,9>)
        n632 = local write "kb"(w1140) -> ()
        n633 = local write "fb_tolerance"(w1146) -> ()
      }
    }
  }
  n634 = while "Sin_wave_gene_p" {
    stop <- FALSE stop-if-true
    n635 = flat-sequence {
      tunnel: [w1215] -> w1175
      tunnel: [w1214] -> w1174
      tunnel: [w1213] -> w1173
      tunnel: [w1212] -> w1172
      tunnel: [w1211] -> w1171
      tunnel: [w1210] -> w1170
      tunnel: [w1209] -> w1169
      tunnel: [w1208] -> w1168
      tunnel: [w1207] -> w1167
      tunnel: [w1193] -> w1166
      tunnel: [w1192] -> w1165
      tunnel: [w1191] -> w1164
      tunnel: [w1190] -> w1163
      tunnel: [w1189] -> w1162
      tunnel: [w1188] -> w1161
      tunnel: [w1187] -> w1160
      tunnel: [w1186] -> w1159
      tunnel: [w1185] -> w1158
      tunnel: [w1179] -> w1157
      tunnel: [w1178] -> w1156
      tunnel: [w1177] -> w1155
      tunnel: w1175 -> [w1266]
      tunnel: w1174 -> [w1265]
      tunnel: w1173 -> [w1264]
      tunnel: w1172 -> [w1263]
      tunnel: w1171 -> [w1262]
      tunnel: w1170 -> [w1261]
      tunnel: w1169 -> [w1260]
      tunnel: w1168 -> [w1259]
      tunnel: w1167 -> [w1258]
      tunnel: w1166 -> [w1251]
      tunnel: w1165 -> [w1246]
      tunnel: w1164 -> [w1242]
      tunnel: w1163 -> [w1250]
      tunnel: w1162 -> [w1245]
      tunnel: w1161 -> [w1241]
      tunnel: w1160 -> [w1249]
      tunnel: w1159 -> [w1243]
      tunnel: w1158 -> [w1240]
      tunnel: w1157 -> [w1230]
      tunnel: w1156 -> [w1229]
      tunnel: w1155 -> [w1228]
      frame #0 {
        n636 = local read "Sin wave time (s)"() -> (w1206:fxp<+,64,32>)
        n637 = local read "Sin wave time (s) b"() -> (w1180:fxp<+,64,32>)
        n638 = call "sin_wave_sub.vi"("Sin_mag"="Sin_mag_p1", "Sin_freq(Hz)"="Sin_freq(Hz)_p1", "Sin wave time (s)"=w1206, "Sin_offset"="Sin_offset_p1", "phase(rad/pi)"="phase(rad/pi)_p1") -> ("Dpr_sin/cos"=w1207:fxp<+/-,22,8>, "Dpr_d"=w1209:fxp<+/-,33,10>, "Dpr_dd"=w1211:fxp<+/-,34,12>)
        n639 = call "sin_wave_sub.vi"("Sin_mag"="Sin_mag_p2", "Sin_freq(Hz)"="Sin_freq(Hz)_p2", "Sin wave time (s)"=w1206, "Sin_offset"="Sin_offset_p2", "phase(rad/pi)"="phase(rad/pi)_p2") -> ("Dpr_sin/cos"=w1208:fxp<+/-,22,8>, "Dpr_d"=w1210:fxp<+/-,33,10>, "Dpr_dd"=w1212:fxp<+/-,34,12>)
        n640 = call "sin_wave_sub.vi"("Sin_mag"="Sin_mag_y1", "Sin_freq(Hz)"="Sin_freq(Hz)_y1", "Sin wave time (s)"=w1206, "Sin_offset"="Sin_offset_y1", "phase(rad/pi)"="phase(rad/pi)_y1") -> ("Dpr_sin/cos"=w1193:fxp<+/-,22,8>, "Dpr_d"=w1192:fxp<+/-,33,10>, "Dpr_dd"=w1191:fxp<+/-,34,12>)
        n641 = call "sin_wave_sub.vi"("Sin_mag"="Sin_mag_y2", "Sin_freq(Hz)"="Sin_freq(Hz)_y2", "Sin wave time (s)"=w1206, "Sin_offset"="Sin_offset_y2", "phase(rad/pi)"="phase(rad/pi)_y2") -> ("Dpr_sin/cos"=w1190:fxp<+/-,22,8>, "Dpr_d"=w1189:fxp<+/-,33,10>, "Dpr_dd"=w1188:fxp<+/-,34,12>)
        n642 = call "sin_wave_sub.vi"("Sin_mag"="Sin_mag_y3", "Sin_freq(Hz)"="Sin_freq(Hz)_y3", "Sin wave time (s)"=w1206, "Sin_offset"="Sin_offset_y3", "phase(rad/pi)"="phase(rad/pi)_y3") -> ("Dpr_sin/cos"=w1187:fxp<+/-,22,8>, "Dpr_d"=w1186:fxp<+/-,33,10>, "Dpr_dd"=w1185:fxp<+/-,34,12>)
        n643 = call "sin_wave_sub.vi"("Sin_mag"="Sin_mag_p3", "Sin_freq(Hz)"="Sin_freq(Hz)_p3", "Sin wave time (s)"=w1206, "Sin_offset"="Sin_offset_p3", "phase(rad/pi)"="phase(rad/pi)_p3") -> ("Dpr_sin/cos"=w1213:fxp<+/-,22,8>, "Dpr_d"=w1214:fxp<+/-,33,10>, "Dpr_dd"=w1215:fxp<+/-,34,12>)
        n644 = call "sin_wave_sub.vi"("Sin_mag"="Sin_mag_b", "Sin_freq(Hz)"="Sin_freq_b (Hz)", "Sin wave time (s)"=w1180, "Sin_offset"="Sin_offset_b", "phase(rad/pi)"="phase(rad/pi)_b") -> ("Dpr_sin/cos"=w1179:fxp<+/-,22,8>, "Dpr_d"=w1178:fxp<+/-,33,10>, "Dpr_dd"=w1177:fxp<+/-,34,12>)
      }
      frame #1 {
        n645 = local read "Step/Sin Db"() -> (w1231:bool)
        n646 = Add(x=w1258, y=w1259) -> (x+y=w1269:fxp<+/-,23,9>)
        n647 = Add(x=w1260, y=w1261) -> (x+y=w1271:fxp<+/-,34,11>)
        n648 = Add(x=w1262, y=w1263) -> (x+y=w1272:fxp<+/-,35,13>)
        n649 = Add(x=w1251, y=w1250) -> (x+y=w1248:fxp<+/-,23,9>)
        n650 = Add(x=w1246, y=w1245) -> (x+y=w1244:fxp<+/-,34,11>)
        n651 = Add(x=w1242, y=w1241) -> (x+y=w1239:fxp<+/-,35,13>)
        n652 = local read "Step/Sin Dpy"() -> (w1236:bool)
        n653 = Add(x=w1248, y=w1249) -> (x+y=→"Dyr_sin/cos":fxp<+/-,24,10>)
        n654 = Add(x=w1244, y=w1243) -> (x+y=w1237:fxp<+/-,35,12>)
        n655 = Add(x=w1239, y=w1240) -> (x+y=w1238:fxp<+/-,36,14>)
        n656 = Add(x=w1269, y=w1264) -> (x+y=→"Dpr_sin/cos":fxp<+/-,24,10>)
        n657 = Add(x=w1271, y=w1265) -> (x+y=w1273:fxp<+/-,35,12>)
        n658 = Add(x=w1272, y=w1266) -> (x+y=w1274:fxp<+/-,36,14>)
        n659 = Select(t=w1229, s=w1231, f=fxp<+/-,33,10> 0.0) -> (s? t:f=→"Dabr_d":fxp<+/-,33,10>)
        n660 = Select(t=w1228, s=w1231, f=fxp<+/-,34,12> 0.0) -> (s? t:f=→"Dabr_dd":fxp<+/-,34,12>)
        n661 = Select(t=w1273, s=w1236, f=fxp<+/-,33,10> 0.0) -> (s? t:f=→"Dpr_d":fxp<+/-,35,12>)
        n662 = Select(t=w1274, s=w1236, f=fxp<+/-,34,12> 0.0) -> (s? t:f=→"Dpr_dd":fxp<+/-,36,14>)
        n663 = Select(t=w1237, s=w1236, f=fxp<+/-,33,10> 0.0) -> (s? t:f=→"Dyr_d":fxp<+/-,35,12>)
        n664 = Select(t=w1238, s=w1236, f=fxp<+/-,34,12> 0.0) -> (s? t:f=→"Dyr_dd":fxp<+/-,36,14>)
        "Dabr_sin/cos" <- w1230
      }
    }
  }
  "Forward/Backward (py)" <- w1
  "Step/Sin Dpy" <- w1
  "Step/Sin Db" <- w2
  "Forward/Backward (b)" <- w2
